vi "Q14070-Z060A - 副本.vi"() -> ()   [LabVIEW 2013]
uses:
  <vilib>/Utility/error.llb/whitespace.ctl
  <vilib>/Utility/file.llb/Read From Spreadsheet File (string).vi
  <vilib>/express/express arith-compare/Formula/XNode/ExpressFormulaBlockNode.xnode
  PCI8622_32.dll
  <vilib>/printing/EasyPrintingControls.llb/contents.ctl
  <vilib>/Utility/NIReport.llb/NI_ReportGenerationCore.lvlib
  <vilib>/printing/EasyPrintingControls.llb/report_type.ctl
  <vilib>/printing/EasyPrinting.llb/Easy Print VI Panel or Documentation (path).vi
  <vilib>/Utility/NIReport.llb/NI_report.lvclass
panel:
  out "最大轴向力标准(N)":dbl=200.0 caption="L+Lmax(mm)" format="%#.3f"
  out "右平均轴向力(N)":dbl caption="L+Lmax(mm)" format="%#.3f"
  out "左平均轴向力(N)":dbl caption="最大位移偏离Lmax(mm)" format="%#.3f"
  out "员工ID":string
  in  "机械间隙值":dbl=2.0
  out "急停":bool
  out "报警":dbl
  out "报警提示":string
  out "DeviceHandle":u32
  in  "设定轴向力调整次数":dbl=6.0
  out "出支线工步号":u32
  in  "最小间隙(mm)":dbl=0.001 format="%#.3f"
  in  "测头气缸右移":bool
  in  "测头气缸左移":bool
  in  "轴向力已做次数":dbl
  out "全行程间隙及轴向力合格":bool
  out "轴向力启动":bool
  out "间隙启动":bool
  in  "夹头松开":bool
  in  "夹头夹紧":bool
  out "找帽扭矩":dbl=8.0 caption="压力传感器" format="%#.2f"
  out "error out":errorcluster
  out "型号数量":i32
  out "error out 4":errorcluster
  in  "设定间隙调整次数":dbl=6.0
  out "读取产品ID":string
  out "下工位备料":bool
  out "下工位测试":bool
  out "下工位自动":bool
  out "下工位备料H":bool
  out "下工位测试H":bool
  out "下工位自动H":bool
  out "FGCS":string
  out "KSJJ":string
  out "Z060ARFID":string
  out "轴向力Y":dbl[](array[numeric])
  out "轴向力X":dbl[](array[numeric])
  out "间隙X数组":dbl[](array[numeric])
  out "间隙Y数组":dbl[](array[numeric])
  out "error out 3":errorcluster caption="错误输出"
  out "rfid工步号":u32
  out "芯片ID":string="201209190001"
  out "rfid完成":bool
  out "rfid触发":bool
  out "本序已做":bool
  in  "回零完成":bool
  in  "电动缸回零":bool
  in  "已调试次数":dbl
  in  "需调整角度(度)":dbl
  in  "转向器中心":dbl
  out "扭矩到达":bool
  out "黄灯":bool
  out "红灯":bool
  in  "基准位移":dbl caption="压力传感器" format="%#.3f"
  out "上序不合格":bool
  out "单点间隙合格":bool
  out "上序合格":bool
  out "测头机构电机":u32
  out "复位":bool
  in  "型号选择":u16(ring)=1 items=["J709", "J728", "J706"]
  in  "联线按钮":bool
  in  "工步号":u32
  in  "产品ID":string="201209190001"
  out "间隙位移(mm)":dbl caption="压力传感器" format="%#.3f"
  out "齿条推拉力(N)":dbl format="%#.2f"
  out "齿条扭矩(Nm)":dbl format="%#.2f"
  out "通讯状态":bool
  in  "员工ID":string
  out "员工姓名":string
  out "工步提示":string
  out "ADODB._Connection Out 2":refnum<k7>
  out "旋转齿条电机":u32
  out "电动缸电机":u32
  in  "停止":bool
  in  "参数加载":bool
  in  "选项卡控件":T1(tab)
  out "扭动曲线":cluster{"Y":dbl[], "Y":dbl[]}[](graph) caption="压球涨堵头1"
  out "中间位置间隙":dbl caption="间隙值L(mm)" format="%#.3f"
  in  "中间间隙标准(mm)":dbl=0.07 format="%#.3f"
  in  "找帽OK":bool
  in  "全行程180°外间隙标准(mm)":dbl=0.1 format="%#.3f"
  out "右180°外全行程间隙":dbl caption="正向最大间隙L1(mm)" format="%#.4f"
  out "左180°外全行程间隙":dbl caption="正向最大间隙L1(mm)" format="%#.4f"
  out "右180°内全行程间隙":dbl caption="正向最大间隙L1(mm)" format="%#.4f"
  out "左180°内全行程间隙":dbl caption="正向最大间隙L1(mm)" format="%#.4f"
  in  "全行程180°内间隙标准(mm)":dbl=0.07 format="%#.3f"
  out "左全行程间隙":dbl caption="正向最大间隙L1(mm)" format="%#.3f"
  out "右全行程间隙":dbl caption="正向最大间隙L1(mm)" format="%#.3f"
  out "总圈数最大值":dbl
  out "总圈数标准":dbl
  out "总行程最大值":dbl
  out "总行程标准(mm)":dbl
  out "平均轴向力MAX(N)":dbl=200.0 caption="L+Lmax(mm)" format="%#.3f"
  out "力波动标准(N)":dbl=60.0 caption="L+Lmax(mm)" format="%#.3f"
  out "轴向力标准(N)":dbl=100.0 caption="L+Lmax(mm)" format="%#.3f"
  out "右最大轴向力(N)":dbl caption="L+Lmax(mm)" format="%#.3f"
  out "左轴向力波动(N)":dbl caption="最大位移偏离Lmax(mm)" format="%#.3f"
  out "左最大轴向力(N)":dbl caption="最大位移偏离Lmax(mm)" format="%#.3f"
  out "行程跳动曲线":cluster{"Y":dbl[], "Y":dbl[]}[](graph) caption="压球涨堵头1"
  out "右轴向力波动(N)":dbl format="%#.3f"
  out "总行程(mm)":dbl format="%#.2f"
  out "总圈数":dbl format="%#.2f"
  in  "不合格品":bool
  in  "扭矩停止值":dbl=16.0
  in  "齿条右极限":dbl=-70.0 caption="压力传感器" format="%#.2f"
  in  "齿条左极限":dbl=-262.0 caption="压力传感器" format="%#.2f"
  in  "齿条移动速度":dbl=5.0 caption="压力传感器" format="%#.2f"
  in  "旋转伺服找帽转速":dbl=5.0 caption="压力传感器" format="%#.2f"
  in  "测量点扭矩":dbl=4.0 caption="压力传感器" format="%#.2f"
  in  "旋转伺服测量转速":dbl caption="压力传感器" format="%#.2f"
  in  "测头机构轴后退位":dbl=30.0 caption="压力传感器" format="%#.2f"
  in  "测头机构轴待检位":dbl caption="压力传感器" format="%#.2f"
  in  "测头机构轴检测位":dbl caption="压力传感器" format="%#.2f"
  in  "测头机构轴移动速度":dbl caption="压力传感器" format="%#.2f"
  in  "全行程修正":dbl=5.5
  out "点胶":bool
  in  "夹头松开":bool
  in  "夹头夹紧":bool
  in  "测头气缸右移":bool
  in  "测头气缸左移":bool
  in  "支线下降":bool
  in  "支线顶升":bool
  in  "出支线":bool
  in  "进支线":bool
  in  "主线下降":bool
  in  "主线顶升":bool
  in  "下阻挡器放行":bool
  in  "上阻挡器放行":bool
  out "夹头夹紧位":bool
  out "测头左位":bool
  out "测头右位":bool
  out "夹头松开":bool
  out "记号笔":bool
  in  "测头机构轴使能":bool
  in  "测头机构轴后退":bool
  in  "测头机构轴前进":bool
  in  "电动缸速度(mm/s)":dbl=10.0 format="%#.3f"
  out "电动缸位置(mm)":dbl=10000.0 format="%#.3f"
  in  "旋转伺服速度(°/s)":dbl=10.0 format="%#.3f"
  out "旋转伺服位置(°)":dbl=10000.0 format="%#.3f"
  in  "测头机构轴速度(mm/s)":dbl=10.0 format="%#.3f"
  out "测头机构轴位置(mm)":dbl=10000.0 format="%#.3f"
  in  "旋转齿条轴右转":bool
  in  "旋转齿条轴左转":bool
  in  "旋转齿条轴使能":bool
  in  "电动缸后退":bool
  in  "电动缸使能":bool
  in  "电动缸前进":bool
  in  "齿条扭矩比例偏移":dbl=1.0 format="%#.2f"
  in  "齿条扭矩零点偏移":dbl format="%#.2f"
  in  "齿条推拉力比例偏移":dbl=1.0 format="%#.2f"
  in  "齿条推拉力零点偏移":dbl format="%#.2f"
  in  "间隙位移比例偏移":dbl=1.0 format="%#.2f"
  in  "间隙位移零点偏移":dbl format="%#.2f"
  in  "传感器参数保存":bool
  in  "参数修改":bool
  in  "参数查询":bool
  in  "参数浏览表":string[][](table)
  # "芜湖机械转向器装配线"
  # "间隙及轴向力检测"
  # "Q14070机械转向器装配线"
  # "湖北唯思凌科装备制造有限公司 设计开发 (C)2015"
  # "≤"
  # "间隙测量判定值"
  # "间隙测量结果"
  # "≤"
  # "≤"
  # "≤"
  # "轴向力测量结果"
  # "轴向力测量标准"
  # "≤"
  # "≥"
  # "≤"
  # "≥"
  # "≤"
  # "≥"
  # "≤"
  # "不得大于20NM"
  # "传感器校验区"
  # "关于传感器校验：\n1、传感器校验需要由具备资质的单位或部门进行校验。\n2、具备权限的用户才能够修改传感器校验参数和试验参数。\n3、修改校验参数方法：先将比例偏移置为1，修改零点偏移，使零点值与校验的传感器一致；然后根据增幅调整比例偏移。"
  # "注意：\n具备权限的用户才能够修改传感器校验参数和试验参数！"
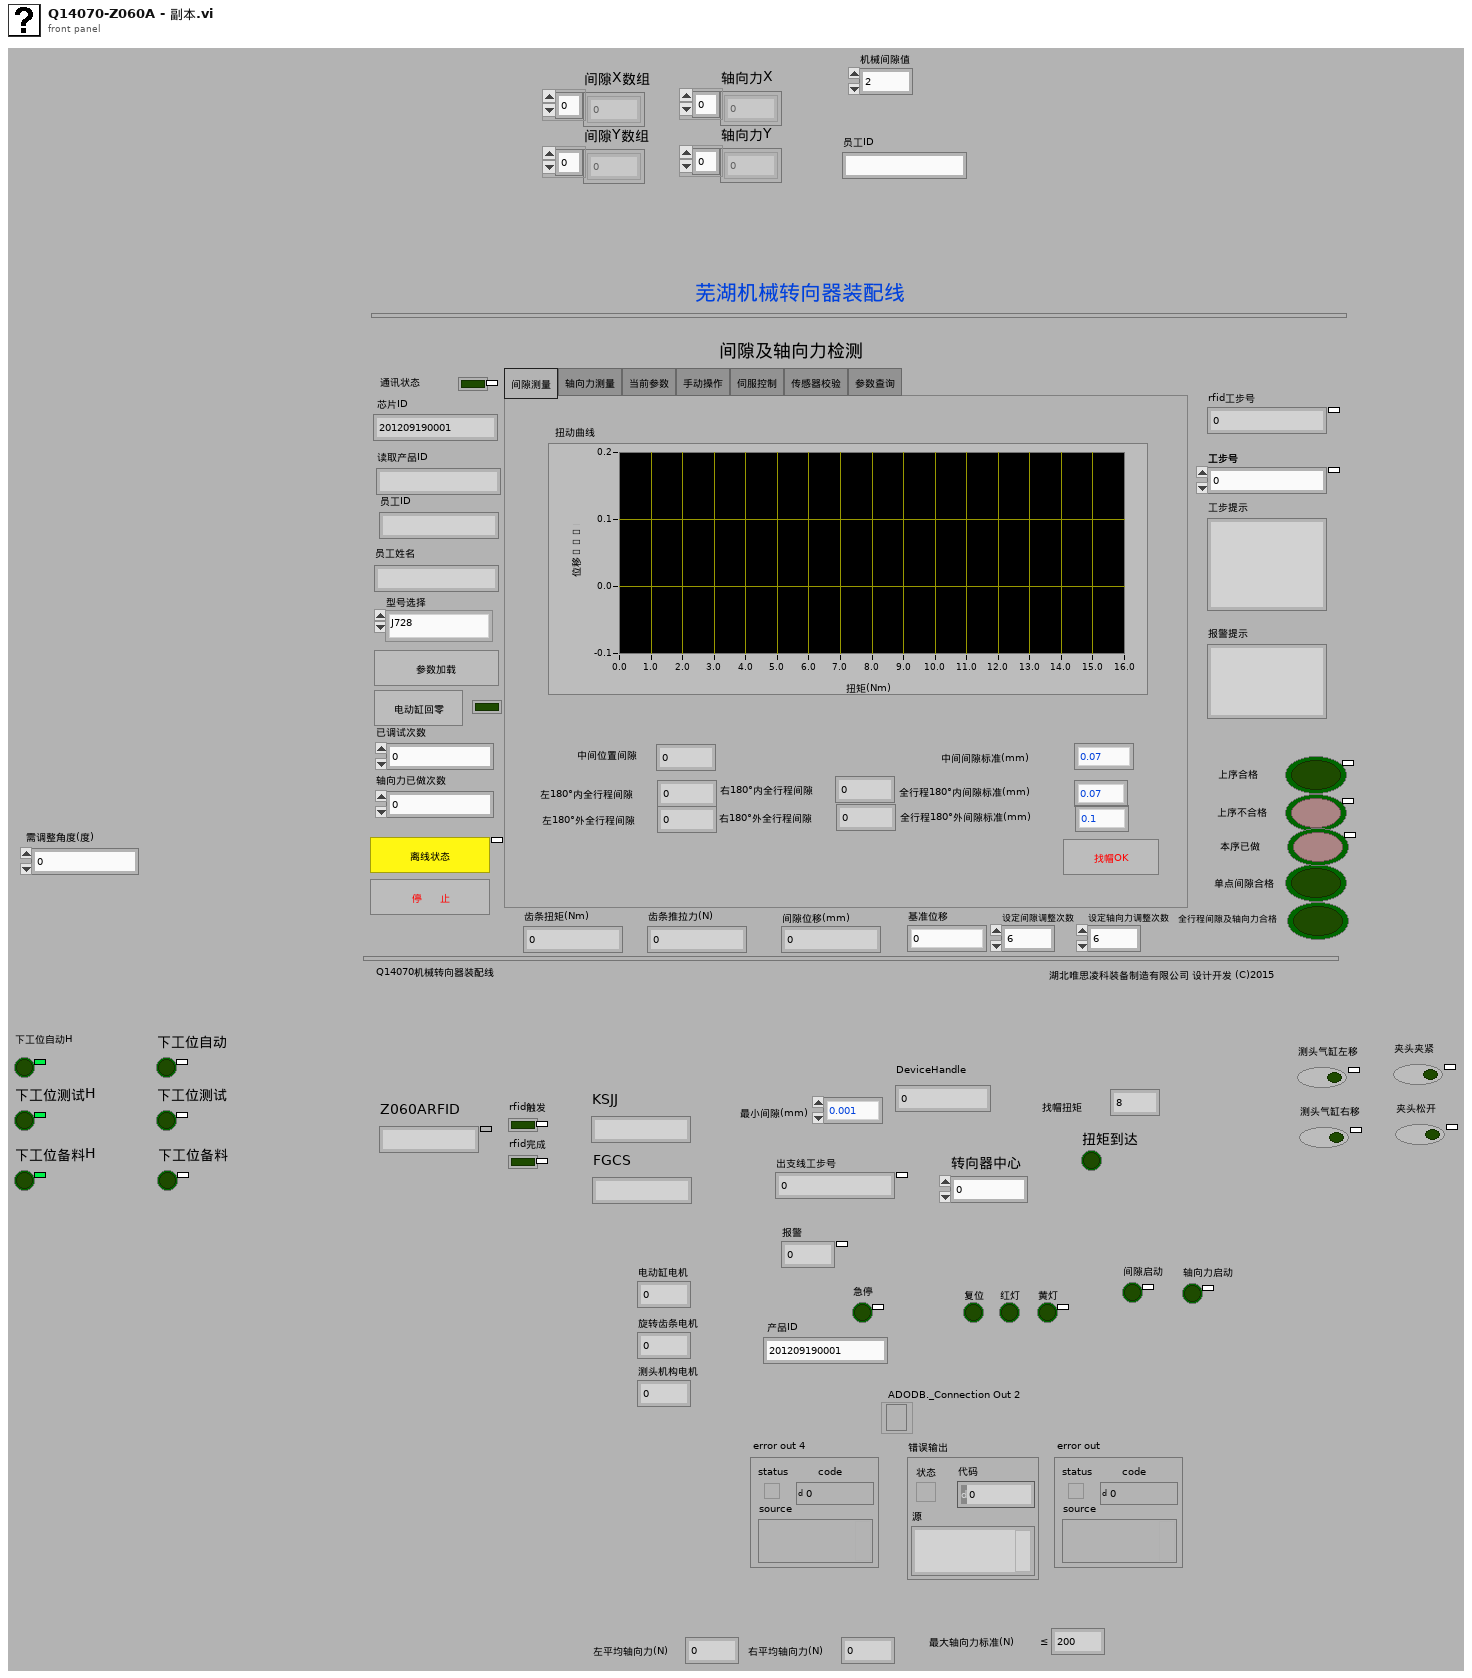
[diagram p1: front panel]
types:
  T1 = enum32{"间隙测量", "轴向力测量", "当前参数", "手动操作", "伺服控制", "传感器校验", "参数查询"}
  T2 = typedef "NI_ReportGenerationCore.lvlib/report_type.ctl" = u16
  T3 = typedef "NI_ReportGenerationCore.lvlib/contents.ctl" = u16
  T4 = typedef "imagedata.ctl" = cluster{"image type":i32, "image depth":i32, "image":u8[], "mask":u8[], "colors":u32[], "Rectangle":cluster{"left":i16, "top":i16, "right":i16, "bottom":i16}}
  T5 = enum8{"Enabled", "Disabled", "Disabled and Grayed Out"}
  T6 = typedef "whitespace.ctl" = u16
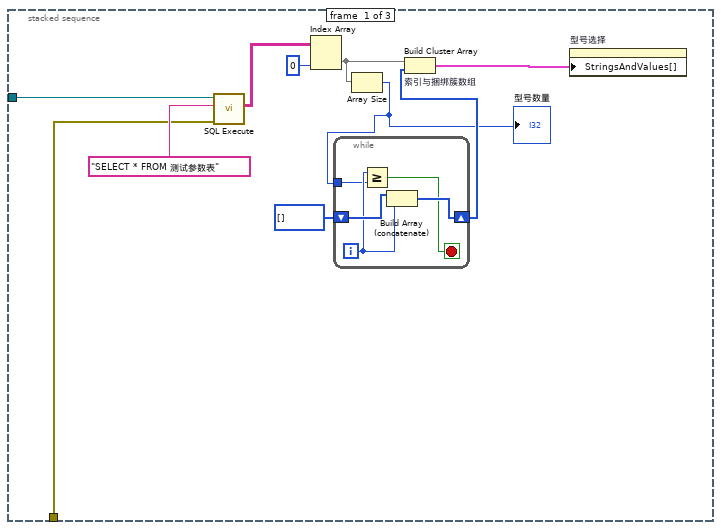
[diagram p4: hidden frame]
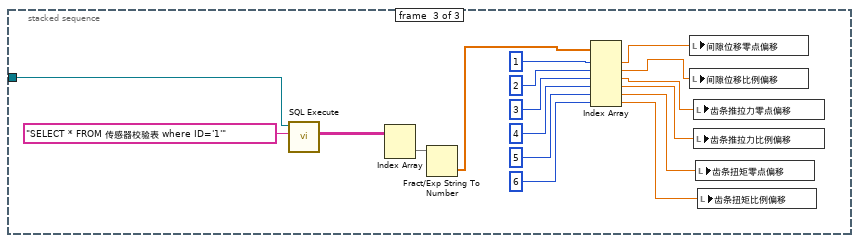
[diagram p5: hidden frame]
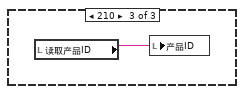
[diagram p7: hidden frame]
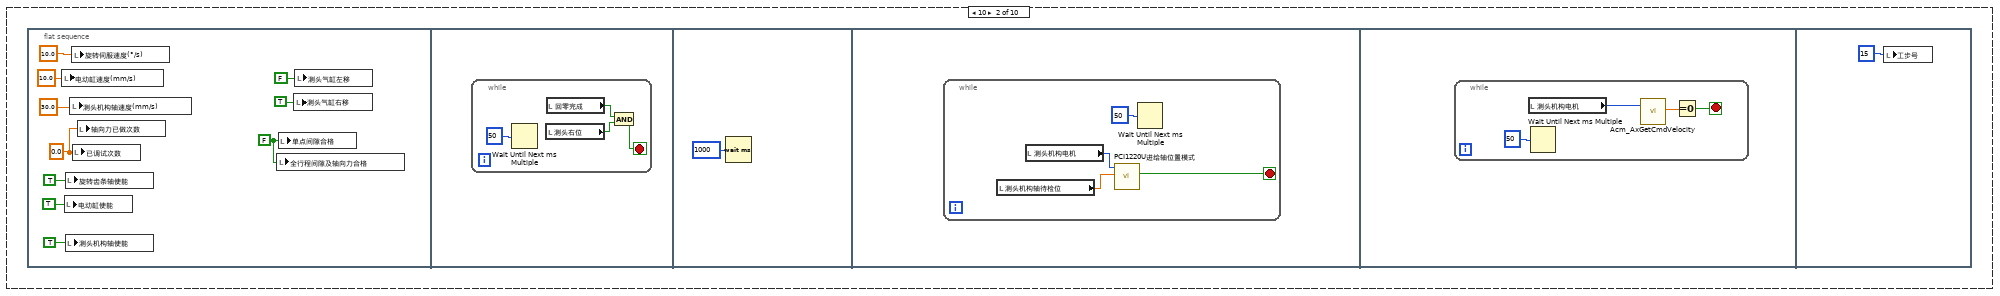
[diagram p9: hidden frame]
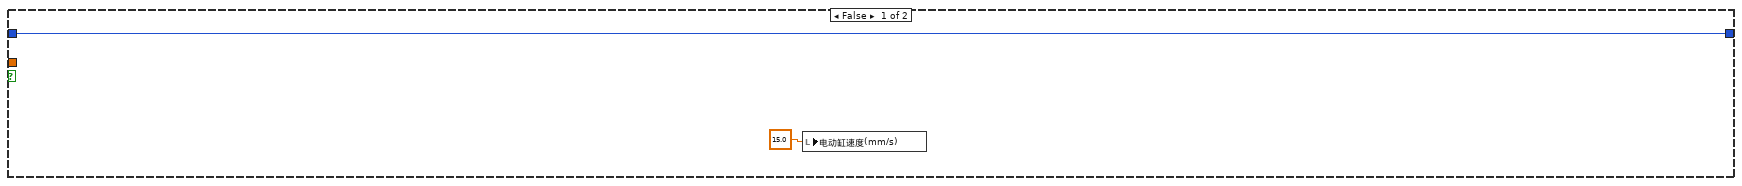
[diagram p10: hidden frame]
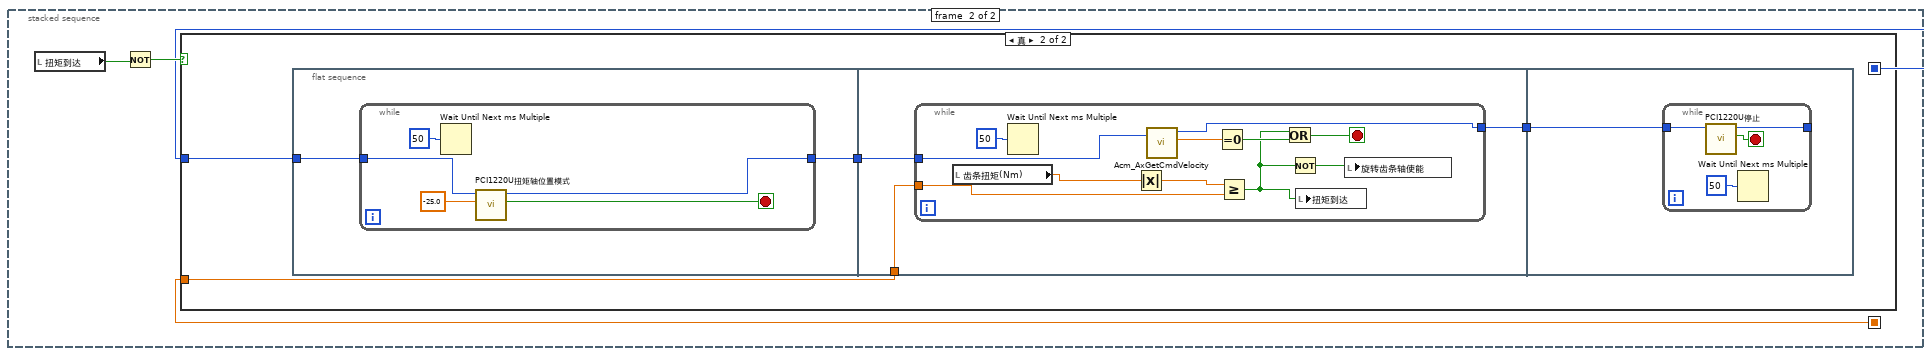
[diagram p11: hidden frame]
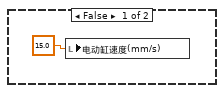
[diagram p12: hidden frame]
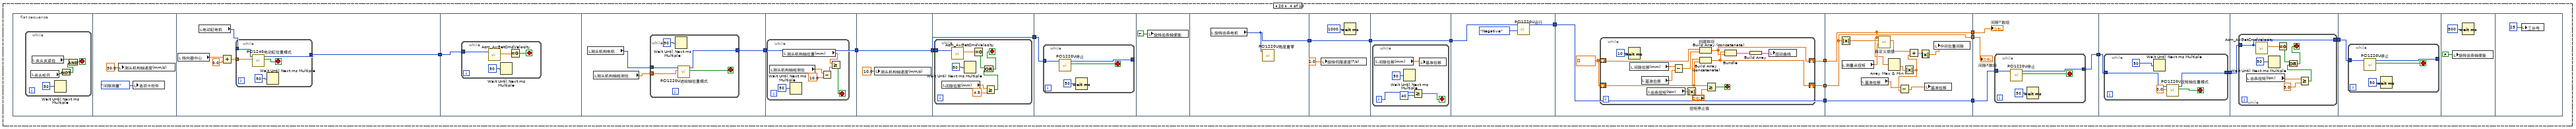
[diagram p14: hidden frame]
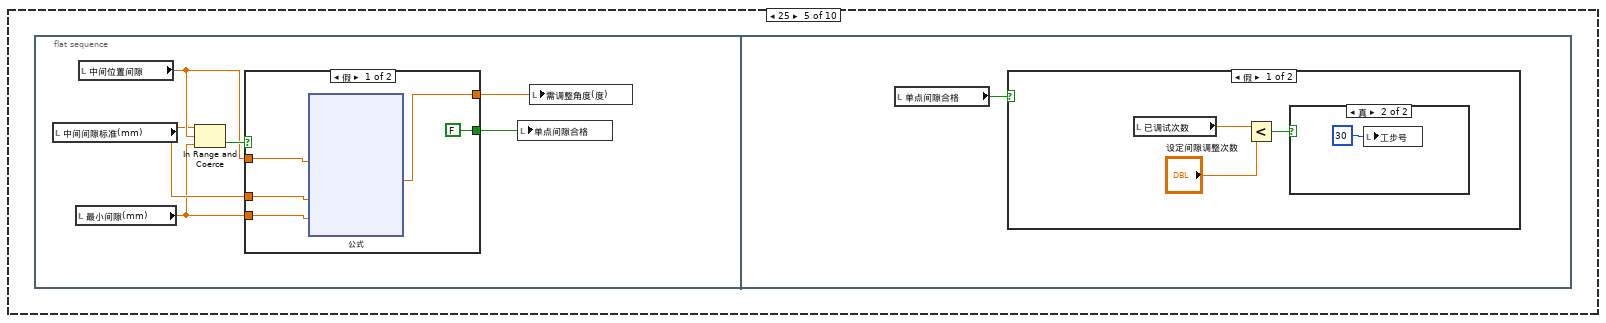
[diagram p15: hidden frame]
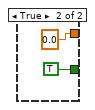
[diagram p16: hidden frame]
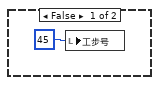
[diagram p17: hidden frame]
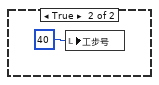
[diagram p18: hidden frame]
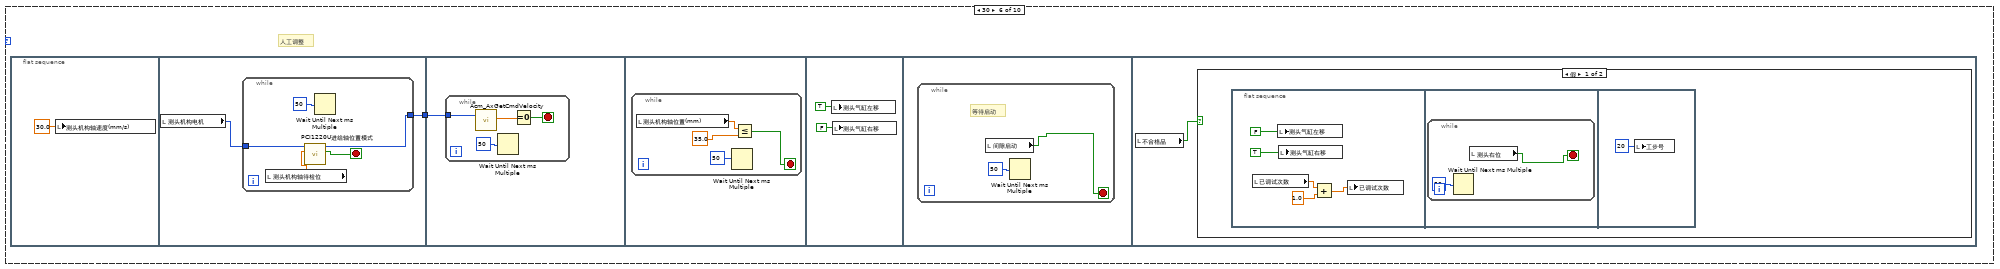
[diagram p19: hidden frame]
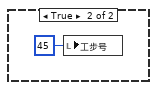
[diagram p20: hidden frame]
diagram:
  n1 = while {
    stop <- w7 stop-if-true
    n2 = local read "工步号"() -> (w5:u32)
    n3 = case shown="15" w5 {
      frame 0, Default {
      }
      frame 10 {
        n4 = flat-sequence {
          frame #0 {
            w8 = FALSE ("单点间隙合格")
            w9 = 0.0 ("已调试次数")
            n5 = local write "电动缸速度(mm/s)"(10.0 ("电动缸速度(mm/s)")) -> ()
            n6 = local write "电动缸使能"(TRUE ("电动缸使能")) -> ()
            n7 = local write "旋转齿条轴使能"(TRUE ("旋转齿条轴使能")) -> ()
            n8 = local write "测头机构轴使能"(TRUE ("调整机构轴使能")) -> ()
            n9 = local write "测头机构轴速度(mm/s)"(30.0 ("调整机构轴速度(mm/s)")) -> ()
            n10 = local write "旋转伺服速度(°/s)"(10.0 ("旋转齿条轴速度(°/s)")) -> ()
            n11 = local write "已调试次数"(w9) -> ()
            n12 = local write "轴向力已做次数"(w9) -> ()
            n13 = local write "全行程间隙及轴向力合格"(w8) -> ()
            n14 = local write "单点间隙合格"(w8) -> ()
            n15 = local write "测头气缸右移"(TRUE ("测头气缸右移")) -> ()
            n16 = local write "测头气缸左移"(FALSE ("测头气缸左移")) -> ()
          }
          frame #1 {
            n17 = while {
              stop <- w18 stop-if-true
              n18 = Wait Until Next ms Multiple(millisecond multiple=u32 50 ("毫秒倍数")) -> ()  [unwired: 1 out]
              n19 = local read "测头右位"() -> (w19:bool)
              n20 = local read "回零完成"() -> (w20:bool)
              n21 = And(x=w20, y=w19) -> (x .and. y?=w18:bool)
            }
          }
          frame #2 {
            n22 = Wait (ms)(milliseconds to wait=u32 1000 ("等待时间（毫秒）")) -> ()  [unwired: 1 out]
          }
          frame #3 {
            n23 = while {
              stop <- w26 stop-if-true
              n24 = local read "测头机构轴待检位"() -> (w23:dbl)
              n25 = local read "测头机构电机"() -> (w24:u32)
              n26 = call "PCI1220U进给轴位置模式.vi"("Distance"=w23, "AxisHandle IN"=w24) -> ("AbsSuccess"=w26:bool)  [unwired: 8 in, 1 out]
              n27 = Wait Until Next ms Multiple(millisecond multiple=u32 50 ("毫秒倍数")) -> ()  [unwired: 1 out]
            }
          }
          frame #4 {
            n28 = while {
              stop <- w29 stop-if-true
              n29 = local read "测头机构电机"() -> (w27:u32)
              n30 = Wait Until Next ms Multiple(millisecond multiple=u32 50 ("毫秒倍数")) -> ()  [unwired: 1 out]
              n31 = call <userlib>:"Acm_AxGetCmdVelocity.vi"("AxisHandle"=w27) -> ("Velocity"=w30:dbl)  [unwired: 1 in, 3 out]
              n32 = Equal To 0?(x=w30) -> (x = 0?=w29:bool)
            }
          }
          frame #5 {
            n33 = local write "工步号"(u32 15 ("工步号")) -> ()
          }
        }
      }
      frame 15 {
        n34 = flat-sequence {
          tunnel: [w42] -> w33
          tunnel: w33 -> [w144]
          tunnel: [w144] -> w34
          tunnel: [w149] -> w37
          tunnel: ["转向器中心"] -> w36
          tunnel: w34 -> [w149]
          tunnel: w37 -> [w158]
          tunnel: w36 -> [w157]
          tunnel: [w156] -> w35
          tunnel: w35 -> [w165]
          tunnel: [w164] -> w32
          tunnel: w32 -> [w176]
          frame #0 {
            n35 = local write "扭矩到达"(FALSE ("扭矩到达")) -> ()
            n36 = local write "旋转伺服速度(°/s)"(10.0 ("旋转齿条轴速度(°/s)")) -> ()
            "找帽扭矩" <- 8.0 ("找帽扭矩")
          }
          frame #1 {
            n37 = Wait Until Next ms Multiple(millisecond multiple=u32 50 ("毫秒倍数")) -> ()  [unwired: 1 out]
            n38 = while {
              stop <- w45 stop-if-true
              n39 = stacked-sequence {
                seq-local: [w47 _] -> [_ w88]
                seq-local: [w51 _] -> [_ w87]
                frame #0 {
                  n40 = local read "扭矩到达"() -> (w49:bool)
                  n41 = local read "找帽扭矩"() -> (w47:dbl)
                  n42 = local read "旋转齿条电机"() -> (w48:u32)
                  n43 = Not(x=w49) -> (.not. x?=w50:bool)
                  n44 = case shown="真" w50 {
                    tunnel: [w53 w54] -> w51
                    tunnel: w48 -> [w53 w58]
                    tunnel: w47 -> [_ w56]
                    frame False {
                      n45 = local write "电动缸速度(mm/s)"(15.0 ("电动缸速度(mm/s)")) -> ()
                    }
                    frame True {
                      n46 = flat-sequence {
                        tunnel: w58 -> [w60]
                        tunnel: [w59] -> w57
                        tunnel: w57 -> [w68]
                        tunnel: w56 -> [w67]
                        tunnel: [w66] -> w55
                        tunnel: w55 -> [w81]
                        tunnel: [w80] -> w54
                        frame #0 {
                          n47 = while {
                            tunnel: [w64] -> w59
                            tunnel: w60 -> [w61]
                            stop <- w63 stop-if-true
                            n48 = Wait Until Next ms Multiple(millisecond multiple=u32 50 ("毫秒倍数")) -> ()  [unwired: 1 out]
                            n49 = call "PCI1220U扭矩轴位置模式.vi"("Distance"=13.0, "AxisHandle IN"=w61) -> ("AbsSuccess"=w63:bool, "AxisHandle OUT"=w64:u32)  [unwired: 8 in]
                          }
                        }
                        frame #1 {
                          n50 = while {
                            tunnel: w68 -> [w78]
                            tunnel: w67 -> [w73]
                            tunnel: [w72] -> w66
                            stop <- w74 stop-if-true
                            n51 = local read "齿条扭矩(Nm)"() -> (w71:dbl)
                            n52 = Wait Until Next ms Multiple(millisecond multiple=u32 10 ("毫秒倍数")) -> ()  [unwired: 1 out]
                            n53 = Absolute Value(x=w71) -> (abs(x)=w76:dbl)
                            n54 = call <userlib>:"Acm_AxGetCmdVelocity.vi"("AxisHandle"=w78) -> ("Velocity"=w77:dbl, "AxisHandle"=w72:u32)  [unwired: 1 in, 2 out]
                            n55 = Equal To 0?(x=w77) -> (x = 0?=w75:bool)
                            n56 = Greater Or Equal?(x=w76, y=w73) -> (x >= y?=w70:bool)
                            n57 = Or "或"(x=w70, y=w75) -> (x .or. y?=w74:bool)
                            n58 = local write "扭矩到达"(w70) -> ()
                            n59 = Not(x=w70) -> (.not. x?=w69:bool)
                            n60 = local write "旋转齿条轴使能"(w69) -> ()
                          }
                        }
                        frame #2 {
                          n61 = while {
                            tunnel: w81 -> [w85]
                            tunnel: [w82] -> w80
                            stop <- w84 stop-if-true
                            n62 = call "PCI1220U停止.vi"("AxisHandle IN"=w85) -> ("完成"=w84:bool, "AxisHandle OUT"=w82:u32)  [unwired: 9 in]
                            n63 = Wait Until Next ms Multiple(millisecond multiple=u32 50 ("毫秒倍数")) -> ()  [unwired: 1 out]
                          }
                        }
                      }
                    }
                  }
                }
                frame #1 {
                  n64 = local read "扭矩到达"() -> (w86:bool)
                  n65 = Not(x=w86) -> (.not. x?=w89:bool)
                  n66 = case shown="真" w89 {
                    tunnel: w87 -> [_ w94]
                    tunnel: w88 -> [_ w92]
                    frame False {
                      n67 = local write "电动缸速度(mm/s)"(15.0 ("电动缸速度(mm/s)")) -> ()
                    }
                    frame True {
                      n68 = flat-sequence {
                        tunnel: w94 -> [w95]
                        tunnel: [w96] -> w93
                        tunnel: w93 -> [w104]
                        tunnel: w92 -> [w103]
                        tunnel: [w102] -> w91
                        tunnel: w91 -> [w116]
                        frame #0 {
                          n69 = while {
                            tunnel: [w100] -> w96
                            tunnel: w95 -> [w97]
                            stop <- w99 stop-if-true
                            n70 = Wait Until Next ms Multiple(millisecond multiple=u32 50 ("毫秒倍数")) -> ()  [unwired: 1 out]
                            n71 = call "PCI1220U扭矩轴位置模式.vi"("Distance"=-25.0, "AxisHandle IN"=w97) -> ("AbsSuccess"=w99:bool, "AxisHandle OUT"=w100:u32)  [unwired: 8 in]
                          }
                        }
                        frame #1 {
                          n72 = while {
                            tunnel: w104 -> [w114]
                            tunnel: [w109] -> w102
                            tunnel: w103 -> [w108]
                            stop <- w110 stop-if-true
                            n73 = local read "齿条扭矩(Nm)"() -> (w107:dbl)
                            n74 = Wait Until Next ms Multiple(millisecond multiple=u32 50 ("毫秒倍数")) -> ()  [unwired: 1 out]
                            n75 = Absolute Value(x=w107) -> (abs(x)=w112:dbl)
                            n76 = call <userlib>:"Acm_AxGetCmdVelocity.vi"("AxisHandle"=w114) -> ("Velocity"=w113:dbl, "AxisHandle"=w109:u32)  [unwired: 1 in, 2 out]
                            n77 = Equal To 0?(x=w113) -> (x = 0?=w111:bool)
                            n78 = Greater Or Equal?(x=w112, y=w108) -> (x >= y?=w105:bool)
                            n79 = Or(x=w105, y=w111) -> (x .or. y?=w110:bool)
                            n80 = Not(x=w105) -> (.not. x?=w106:bool)
                            n81 = local write "扭矩到达"(w105) -> ()
                            n82 = local write "旋转齿条轴使能"(w106) -> ()
                          }
                        }
                        frame #2 {
                          n83 = while {
                            tunnel: w116 -> [w120]
                            tunnel: [w117] -> _
                            stop <- w119 stop-if-true
                            n84 = call "PCI1220U停止.vi"("AxisHandle IN"=w120) -> ("完成"=w119:bool, "AxisHandle OUT"=w117:u32)  [unwired: 9 in]
                            n85 = Wait Until Next ms Multiple(millisecond multiple=u32 50 ("毫秒倍数")) -> ()  [unwired: 1 out]
                          }
                        }
                      }
                    }
                  }
                }
              }
              n86 = Wait Until Next ms Multiple(millisecond multiple=u32 50 ("毫秒倍数")) -> ()  [unwired: 1 out]
              n87 = local read "扭矩到达"() -> (w45:bool)
            }
            n88 = flat-sequence {
              tunnel: [w122] -> w44
              tunnel: w44 -> [w128]
              tunnel: [w128] -> w41
              tunnel: [w137] -> w42
              tunnel: w41 -> [w137]
              frame #0 {
                n89 = local write "电动缸速度(mm/s)"(5.0 ("电动缸速度(mm/s)")) -> ()
              }
              frame #1 {
                n90 = while {
                  tunnel: [w126] -> w122
                  stop <- w125 stop-if-true
                  n91 = local read "齿条左极限"() -> (w123:dbl)
                  n92 = local read "电动缸电机"() -> (w127:u32)
                  n93 = Wait Until Next ms Multiple(millisecond multiple=u32 50 ("毫秒倍数")) -> ()  [unwired: 1 out]
                  n94 = call "PCI1240电动缸位置模式 .vi"("Distance"=w123, "AxisHandle IN"=w127) -> ("AbsSuccess"=w125:bool, "AxisHandle OUT"=w126:u32)  [unwired: 8 in]
                }
              }
              frame #2 {
                n95 = while {
                  tunnel: w128 -> [w135]
                  stop <- w132 stop-if-true
                  n96 = local read "齿条推拉力(N)"() -> (w131:dbl)
                  n97 = call <userlib>:"Acm_AxGetCmdVelocity.vi"("AxisHandle"=w135) -> ("Velocity"=w136:dbl)  [unwired: 1 in, 3 out]
                  n98 = Wait Until Next ms Multiple(millisecond multiple=u32 50 ("毫秒倍数")) -> ()  [unwired: 1 out]
                  n99 = Less Or Equal?(x=w131, y=-1000.0) -> (x <= y?=w129:bool)
                  n100 = Equal To 0?(x=w136) -> (x = 0?=w133:bool)
                  n101 = Or(x=w133, y=w129) -> (x .or. y?=w132:bool)
                }
              }
              frame #3 {
                n102 = while {
                  tunnel: w137 -> [w141]
                  tunnel: [w138] -> _
                  stop <- w140 stop-if-true
                  n103 = call "PCI1220U停止.vi"("AxisHandle IN"=w141) -> ("完成"=w140:bool, "AxisHandle OUT"=w138:u32)  [unwired: 9 in]
                  n104 = Wait Until Next ms Multiple(millisecond multiple=u32 50 ("毫秒倍数")) -> ()  [unwired: 1 out]
                }
              }
            }
          }
          frame #2 {
            n105 = while {
              stop <- "找帽OK" stop-if-true
              n106 = Wait Until Next ms Multiple(millisecond multiple=u32 50 ("毫秒倍数")) -> ()  [unwired: 1 out]
            }
            n107 = Wait Until Next ms Multiple(millisecond multiple=u32 500 ("毫秒倍数")) -> ()  [unwired: 1 out]
            n108 = local write "夹头夹紧"(TRUE ("夹头夹紧")) -> ()
            n109 = local write "夹头松开"(FALSE ("夹头松开")) -> ()
          }
          frame #3 {
            n110 = disable-structure shown="禁用" {
              disable-tunnel: [w153 _] -> _
              frame Disabled {
                n111 = local read "齿条右极限"() -> (w151:dbl)
                n112 = local read "齿条左极限"() -> (w152:dbl)
                n113 = Add(x=w152, y=w151) -> (x+y=w155:dbl)
                n114 = Divide(x=w155, y=2.0) -> (x/y=w153:dbl)
              }
              frame Enabled {
              }
            }
            n115 = local write "电动缸速度(mm/s)"(15.0 ("电动缸轴移动速度")) -> ()
          }
          frame #4 {
            n116 = while {
              tunnel: w158 -> [w163]
              tunnel: w157 -> [w162]
              tunnel: [w159] -> w156
              stop <- w161 stop-if-true
              n117 = call "PCI1240电动缸位置模式 .vi"("Distance"=w162, "AxisHandle IN"=w163) -> ("AbsSuccess"=w161:bool, "AxisHandle OUT"=w159:u32)  [unwired: 8 in]
              n118 = Wait Until Next ms Multiple(millisecond multiple=u32 50 ("毫秒倍数")) -> ()  [unwired: 1 out]
            }
          }
          frame #5 {
            n119 = while {
              tunnel: w165 -> [w175]
              tunnel: [w166] -> w164
              stop <- w167 stop-if-true
              n120 = local read "齿条推拉力(N)"() -> (w172:dbl)
              n121 = call <userlib>:"Acm_AxGetCmdVelocity.vi"("AxisHandle"=w175) -> ("Velocity"=w174:dbl, "AxisHandle"=w166:u32)  [unwired: 1 in, 2 out]
              n122 = Wait Until Next ms Multiple(millisecond multiple=u32 50 ("毫秒倍数")) -> ()  [unwired: 1 out]
              n123 = Equal To 0?(x=w174) -> (x = 0?=w169:bool)
              n124 = Absolute Value(x=w172) -> (abs(x)=w171:dbl)
              n125 = Greater Or Equal?(x=w171, y=1000.0) -> (x >= y?=w168:bool)
              n126 = Or(x=w169, y=w168) -> (x .or. y?=w167:bool)
            }
          }
          frame #6 {
            n127 = while {
              tunnel: w176 -> [w180]
              tunnel: [w179] -> _
              stop <- w178 stop-if-true
              n128 = call "PCI1220U停止.vi"("AxisHandle IN"=w180) -> ("完成"=w178:bool, "AxisHandle OUT"=w179:u32)  [unwired: 9 in]
              n129 = Wait (ms)(milliseconds to wait=u32 50 ("毫秒倍数")) -> ()  [unwired: 1 out]
            }
          }
          frame #7 {
            n130 = local write "工步号"(u32 20 ("工步号")) -> ()
          }
        }
      }
      frame 20 {
        n131 = flat-sequence {
          tunnel: [w211] -> w192
          tunnel: w192 -> [w217]
          tunnel: [w223] -> w184
          tunnel: w184 -> [w230]
          tunnel: [w230] -> w183
          tunnel: w183 -> [w238]
          tunnel: [w238] -> w182
          tunnel: w182 -> [w239]
          tunnel: [w239] -> w191
          tunnel: w191 -> [w248]
          tunnel: [w254] -> w189
          tunnel: [w256] -> w190
          tunnel: w189 -> [w256]
          tunnel: [w258] -> w185
          tunnel: w190 -> [w258]
          tunnel: w185 -> [w265]
          tunnel: [w264] -> w196
          tunnel: [w269] -> w195
          tunnel: [w268] -> w194
          tunnel: w196 -> [w267]
          tunnel: [w267] -> w193
          tunnel: [w296] -> w199
          tunnel: [w293] -> w198
          tunnel: w195 -> [w293]
          tunnel: [w292] -> w197
          tunnel: w194 -> [w292]
          tunnel: w193 -> [w296]
          tunnel: w199 -> [w300]
          tunnel: [w299] -> w188
          tunnel: w198 -> [w297]
          tunnel: w197 -> [w298]
          tunnel: w188 -> [w306]
          tunnel: [w305] -> w187
          tunnel: w187 -> [w313]
          tunnel: [w312] -> w186
          tunnel: w186 -> [w322]
          frame #0 {
            n132 = while {
              stop <- w202 stop-if-true
              n133 = local read "夹头松开"() -> (w203:bool)
              n134 = local read "夹头夹紧位"() -> (w201:bool)
              n135 = Wait Until Next ms Multiple(millisecond multiple=u32 50 ("毫秒倍数")) -> ()  [unwired: 1 out]
              n136 = Not(x=w203) -> (.not. x?=w200:bool)
              n137 = And(x=w201, y=w200) -> (x .and. y?=w202:bool)
            }
          }
          frame #1 {
            n138 = local write "测头机构轴速度(mm/s)"(30.0 ("测头机构轴速度(mm/s)")) -> ()
            n139 = local write "选项卡控件"(T1."间隙测量" ("选项卡控件")) -> ()
          }
          frame #2 {
            n140 = local read "转向器中心"() -> (w209:dbl)
            n141 = local read "电动缸电机"() -> (w210:u32)
            n142 = Add(x=w209, y=0.0) -> (x+y=w208:dbl)
            n143 = while {
              tunnel: w210 -> [w216]
              tunnel: w208 -> [w215]
              tunnel: [w212] -> w211
              stop <- w214 stop-if-true
              n144 = call "PCI1240电动缸位置模式 .vi"("Distance"=w215, "AxisHandle IN"=w216) -> ("AbsSuccess"=w214:bool, "AxisHandle OUT"=w212:u32)  [unwired: 8 in]
              n145 = Wait Until Next ms Multiple(millisecond multiple=u32 50 ("毫秒倍数")) -> ()  [unwired: 1 out]
            }
          }
          frame #3 {
            n146 = while {
              tunnel: w217 -> [w221]
              stop <- w219 stop-if-true
              n147 = call <userlib>:"Acm_AxGetCmdVelocity.vi"("AxisHandle"=w221) -> ("Velocity"=w220:dbl)  [unwired: 1 in, 3 out]
              n148 = Wait Until Next ms Multiple(millisecond multiple=u32 50 ("毫秒倍数")) -> ()  [unwired: 1 out]
              n149 = Equal To 0?(x=w220) -> (x = 0?=w219:bool)
            }
          }
          frame #4 {
            n150 = local read "测头机构电机"() -> (w224:u32)
            n151 = local read "测头机构轴检测位"() -> (w222:dbl)
            n152 = while {
              tunnel: w224 -> [w227]
              tunnel: w222 -> [w226]
              tunnel: [w225] -> w223
              stop <- w229 stop-if-true
              n153 = Wait Until Next ms Multiple(millisecond multiple=u32 50 ("毫秒倍数")) -> ()  [unwired: 1 out]
              n154 = call "PCI1220U进给轴位置模式.vi"("Distance"=w226, "AxisHandle IN"=w227) -> ("AbsSuccess"=w229:bool, "AxisHandle OUT"=w225:u32)  [unwired: 8 in]
            }
          }
          frame #5 {
            n155 = while {
              stop <- w231 stop-if-true
              n156 = local read "测头机构轴检测位"() -> (w235:dbl)
              n157 = local read "测头机构轴位置(mm)"() -> (w234:dbl)
              n158 = Wait Until Next ms Multiple(millisecond multiple=u32 50 ("毫秒倍数")) -> ()  [unwired: 1 out]
              n159 = Subtract(x=w235, y=10.0) -> (x-y=w232:dbl)
              n160 = Greater Or Equal?(x=w234, y=w232) -> (x >= y?=w231:bool)
            }
          }
          frame #6 {
            n161 = local write "测头机构轴速度(mm/s)"(10.0 ("测头机构轴速度(mm/s)")) -> ()
          }
          frame #7 {
            n162 = while {
              tunnel: w239 -> [w247]
              stop <- w241 stop-if-true
              n163 = local read "间隙位移(mm)"() -> (w244:dbl)
              n164 = call <userlib>:"Acm_AxGetCmdVelocity.vi"("AxisHandle"=w247) -> ("Velocity"=w246:dbl)  [unwired: 1 in, 3 out]
              n165 = Wait Until Next ms Multiple(millisecond multiple=u32 50 ("毫秒倍数")) -> ()  [unwired: 1 out]
              n166 = Equal To 0?(x=w246) -> (x = 0?=w242:bool)
              n167 = Greater Or Equal?(x=w244, y=4.5) -> (x >= y?=w240:bool)
              n168 = Or(x=w242, y=w240) -> (x .or. y?=w241:bool)
            }
          }
          frame #8 {
            n169 = while {
              tunnel: w248 -> [w252]
              tunnel: [w251] -> _
              stop <- w250 stop-if-true
              n170 = call "PCI1220U停止.vi"("AxisHandle IN"=w252) -> ("完成"=w250:bool, "AxisHandle OUT"=w251:u32)  [unwired: 9 in]
              n171 = Wait (ms)(milliseconds to wait=u32 50 ("毫秒倍数")) -> ()  [unwired: 1 out]
            }
          }
          frame #9 {
            n172 = local write "旋转齿条轴使能"(TRUE ("旋转齿条轴使能")) -> ()
          }
          frame #10 {
            n173 = local read "旋转齿条电机"() -> (w254:u32)
            n174 = call "PCI1220U角度置零.vi"("AxisHandle IN"=w254) -> ()  [unwired: 10 in, 1 out]
          }
          frame #11 {
            n175 = local write "旋转伺服速度(°/s)"(1.0 ("旋转齿条轴速度(°/s)")) -> ()
            n176 = Wait (ms)(milliseconds to wait=u32 1000 ("毫秒倍数")) -> ()  [unwired: 1 out]
          }
          frame #12 {
            n177 = while {
              i -> [w262]
              stop <- w259 stop-if-true
              n178 = local read "间隙位移(mm)"() -> (w263:dbl)
              n179 = Wait Until Next ms Multiple(millisecond multiple=u32 50 ("毫秒倍数")) -> ()  [unwired: 1 out]
              n180 = Greater Or Equal?(x=w262, y=40) -> (x >= y?=w259:bool)
              n181 = local write "基准位移"(w263) -> ()
            }
          }
          frame #13 {
            n182 = call "PCI1220U运行.vi"("方向"=enum32{"Negative", "Positive"}."Negative" ("Direction"), "AxisHandle IN"=w265) -> ("AxisHandle OUT"=w264:u32)  [unwired: 9 in]
          }
          frame #14 {
            w270 = dbl[] []
            n183 = while {
              shift-right: [w281] -> w269
              shift-left: w270 -> [w283]
              shift-right: [w280] -> w268
              shift-left: w270 -> [w282]
              stop <- w273 stop-if-true
              n184 = Wait (ms)(milliseconds to wait=u32 10 ("毫秒倍数")) -> ()  [unwired: 1 out]
              n185 = local read "间隙位移(mm)"() -> (w276:dbl)
              n186 = local read "基准位移"() -> (w274:dbl)
              n187 = local read "齿条扭矩(Nm)"() -> (w277:dbl)
              n188 = Subtract(x=w276, y=w274) -> (x-y=w275:dbl)
              n189 = Absolute Value(x=w277) -> (abs(x)=w272:dbl)
              n190 = Build Array (concatenate) "创建数组"(w282, w275) -> (w280:dbl[])
              n191 = Build Array (concatenate) ("创建数组")(w283, w272) -> (w281:dbl[])
              n192 = Greater Or Equal?(x=w272, y="扭矩停止值") -> (x >= y?=w273:bool)
              n193 = Bundle ("捆绑")(w281, w280) -> (w278:cluster{dbl[], dbl[]})  [unwired: 1 in]
              n194 = Build Array ("创建数组")(w278) -> (w279:cluster{dbl[], dbl[]}[])
              n195 = local write "扭动曲线"(w279) -> ()
            }
          }
          frame #15 {
            n196 = Absolute Value(x=w293) -> (abs(x)=w294:dbl[])
            n197 = local read "测量点扭矩"() -> (w295:dbl)
            n198 = local read "基准位移"() -> (w289:dbl)
            n199 = call "自定义插值.vi"("压力"=w295, "扭矩数组"=w294, "位移数组"=w292) -> ("扭矩值"=w290:dbl)  [unwired: 8 in]
            n200 = Array Max & Min(array=w292) -> (min value=w291:dbl)  [unwired: 3 out]
            n201 = Absolute Value(x=w291) -> (abs(x)=w288:dbl)
            n202 = Subtract(x=w289, y=w288) -> (x-y=w287:dbl)
            n203 = Add(x=w290, y=w288) -> (x+y=w286:dbl)
            n204 = Absolute Value(x=w286) -> (abs(x)=w285:dbl)
            n205 = local write "基准位移"(w287) -> ()
            n206 = local write "中间位置间隙"(w285) -> ()
          }
          frame #16 {
            n207 = while {
              tunnel: w300 -> [w304]
              tunnel: [w303] -> w299
              stop <- w302 stop-if-true
              n208 = call "PCI1220U停止.vi"("AxisHandle IN"=w304) -> ("完成"=w302:bool, "AxisHandle OUT"=w303:u32)  [unwired: 9 in]
              n209 = Wait (ms)(milliseconds to wait=u32 50 ("毫秒倍数")) -> ()  [unwired: 1 out]
            }
            "间隙Y数组" <- w298
            "间隙X数组" <- w297
          }
          frame #17 {
            n210 = while {
              tunnel: [w311] -> w305
              tunnel: w306 -> [w308]
              stop <- w310 stop-if-true
              n211 = Wait Until Next ms Multiple(millisecond multiple=u32 50 ("毫秒倍数")) -> ()  [unwired: 1 out]
              n212 = call "PCI1220U扭矩轴位置模式.vi"("Distance"=0.0, "AxisHandle IN"=w308) -> ("AbsSuccess"=w310:bool, "AxisHandle OUT"=w311:u32)  [unwired: 8 in]
            }
          }
          frame #18 {
            n213 = while {
              tunnel: w313 -> [w315]
              tunnel: [w315] -> w312
              stop <- w318 stop-if-true
              n214 = local read "齿条扭矩(Nm)"() -> (w314:dbl)
              n215 = call <userlib>:"Acm_AxGetCmdVelocity.vi"("AxisHandle"=w315) -> ("Velocity"=w321:dbl)  [unwired: 1 in, 3 out]
              n216 = Wait Until Next ms Multiple(millisecond multiple=u32 50 ("毫秒倍数")) -> ()  [unwired: 1 out]
              n217 = Equal To 0?(x=w321) -> (x = 0?=w319:bool)
              n218 = Greater Or Equal?(x=w314, y=3.0) -> (x >= y?=w316:bool)
              n219 = Or(x=w319, y=w316) -> (x .or. y?=w318:bool)
            }
          }
          frame #19 {
            n220 = while {
              tunnel: w322 -> [w326]
              tunnel: [w325] -> _
              stop <- w324 stop-if-true
              n221 = call "PCI1220U停止.vi"("AxisHandle IN"=w326) -> ("完成"=w324:bool, "AxisHandle OUT"=w325:u32)  [unwired: 9 in]
              n222 = Wait (ms)(milliseconds to wait=u32 50 ("毫秒倍数")) -> ()  [unwired: 1 out]
            }
          }
          frame #20 {
            n223 = local write "旋转齿条轴使能"(FALSE ("旋转齿条轴使能")) -> ()
            n224 = Wait (ms)(milliseconds to wait=u32 500 ("毫秒倍数")) -> ()  [unwired: 1 out]
          }
          frame #21 {
            n225 = local write "工步号"(u32 25 ("工步号")) -> ()
          }
        }
      }
      frame 25 {
        n226 = flat-sequence {
          frame #0 {
            n227 = local read "中间间隙标准(mm)"() -> (w331:dbl)
            n228 = local read "最小间隙(mm)"() -> (w330:dbl)
            n229 = local read "中间位置间隙"() -> (w332:dbl)
            n230 = In Range and Coerce(upper limit=w331, x=w332, lower limit=w330) -> (In Range?=w335:bool)  [unwired: 1 out]
            n231 = case shown="假" w335 {
              tunnel: [FALSE ("本序合格") TRUE ("本序合格")] -> w334
              tunnel: [w340 0.0 ("需调整角度(度)")] -> w333
              tunnel: w332 -> [w338 _]
              tunnel: w331 -> [w337 _]
              tunnel: w330 -> [w336 _]
              frame False {
                n232 = xnode "公式"("X"=w338, "Xmax"=w337, "Xmin"=w336) -> ("结果"=w340:dbl)  [unwired: 1 in, 1 out]
              }
              frame True {
              }
            }
            n233 = local write "单点间隙合格"(w334) -> ()
            n234 = local write "需调整角度(度)"(w333) -> ()
          }
          frame #1 {
            n235 = local read "单点间隙合格"() -> (w355:bool)
            n236 = case shown="假" w355 {
              frame False {
                n237 = local read "已调试次数"() -> (w358:dbl)
                n238 = Less?(x=w358, y="设定间隙调整次数") -> (x < y?=w357:bool)
                n239 = case shown="真" w357 {
                  frame False {
                    n240 = local write "工步号"(u32 45 ("变更工步号")) -> ()
                  }
                  frame True {
                    n241 = local write "工步号"(u32 30 ("变更工步号")) -> ()
                  }
                }
              }
              frame True {
                n242 = local write "工步号"(u32 40 ("变更工步号")) -> ()
              }
            }
          }
        }
      }
      frame 30 {
        # "人工调整"
        n243 = flat-sequence {
          tunnel: [w364] -> w362
          tunnel: w362 -> [w371]
          frame #0 {
            n244 = local write "测头机构轴速度(mm/s)"(30.0 ("测头机构轴速度(mm/s)")) -> ()
          }
          frame #1 {
            n245 = local read "测头机构电机"() -> (w365:u32)
            n246 = while {
              tunnel: w365 -> [w368]
              tunnel: [w367] -> w364
              stop <- w370 stop-if-true
              n247 = local read "测头机构轴待检位"() -> (w366:dbl)
              n248 = call "PCI1220U进给轴位置模式.vi"("Distance"=w366, "AxisHandle IN"=w368) -> ("AbsSuccess"=w370:bool, "AxisHandle OUT"=w367:u32)  [unwired: 8 in]
              n249 = Wait Until Next ms Multiple(millisecond multiple=u32 50 ("毫秒倍数")) -> ()  [unwired: 1 out]
            }
          }
          frame #2 {
            n250 = while {
              tunnel: w371 -> [w375]
              stop <- w373 stop-if-true
              n251 = call <userlib>:"Acm_AxGetCmdVelocity.vi"("AxisHandle"=w375) -> ("Velocity"=w374:dbl)  [unwired: 1 in, 3 out]
              n252 = Wait Until Next ms Multiple(millisecond multiple=u32 50 ("毫秒倍数")) -> ()  [unwired: 1 out]
              n253 = Equal To 0?(x=w374) -> (x = 0?=w373:bool)
            }
          }
          frame #3 {
            n254 = while {
              stop <- w377 stop-if-true
              n255 = local read "测头机构轴位置(mm)"() -> (w379:dbl)
              n256 = Wait Until Next ms Multiple(millisecond multiple=u32 50 ("毫秒倍数")) -> ()  [unwired: 1 out]
              n257 = Less Or Equal?(x=w379, y=35.0) -> (x <= y?=w377:bool)
            }
          }
          frame #4 {
            n258 = local write "测头气缸左移"(TRUE ("测头气缸左移")) -> ()
            n259 = local write "测头气缸右移"(FALSE ("测头气缸右移")) -> ()
          }
          frame #5 {
            n260 = while {
              stop <- w382 stop-if-true
              # "等待启动"
              n261 = local read "间隙启动"() -> (w382:bool)
              n262 = Wait Until Next ms Multiple(millisecond multiple=u32 50 ("毫秒倍数")) -> ()  [unwired: 1 out]
            }
          }
          frame #6 {
            n263 = local read "不合格品"() -> (w384:bool)
            n264 = case shown="假" w384 {
              frame False {
                n265 = flat-sequence {
                  frame #0 {
                    n266 = local read "已调试次数"() -> (w387:dbl)
                    n267 = local write "测头气缸左移"(FALSE ("测头气缸左移")) -> ()
                    n268 = local write "测头气缸右移"(TRUE ("测头气缸左移")) -> ()
                    n269 = Add(x=w387, y=1.0 ("已调试次数")) -> (x+y=w389:dbl)
                    n270 = local write "已调试次数"(w389) -> ()
                  }
                  frame #1 {
                    n271 = while {
                      stop <- w390 stop-if-true
                      n272 = Wait Until Next ms Multiple(millisecond multiple=u32 50 ("毫秒倍数")) -> ()  [unwired: 1 out]
                      n273 = local read "测头右位"() -> (w390:bool)
                    }
                  }
                  frame #2 {
                    n274 = local write "工步号"(u32 20 ("工步号")) -> ()
                  }
                }
              }
              frame True {
                n275 = local write "工步号"(u32 45 ("工步号")) -> ()
              }
            }
          }
        }
      }
      frame 40 {
        n276 = flat-sequence {
          tunnel: [w492] -> w488
          tunnel: w488 -> [w494]
          tunnel: [w493] -> w486
          tunnel: w486 -> [w500]
          tunnel: [w500] -> w471
          tunnel: w471 -> [w509]
          tunnel: [w509] -> w470
          tunnel: w470 -> [w516]
          tunnel: [w516] -> w485
          tunnel: w485 -> [w518]
          tunnel: [w519] -> w469
          tunnel: [w517] -> w468
          tunnel: [w531] -> w478
          tunnel: [w530] -> w477
          tunnel: [w529] -> w476
          tunnel: w469 -> [w528]
          tunnel: [w528] -> w475
          tunnel: [w526] -> w473
          tunnel: w468 -> [w525]
          tunnel: w478 -> [w571]
          tunnel: [w571] -> w445
          tunnel: w477 -> [w578]
          tunnel: [w578] -> w443
          tunnel: w476 -> [w574]
          tunnel: [w574] -> w441
          tunnel: w475 -> [w577]
          tunnel: [w577] -> w439
          tunnel: [w573] -> w437
          tunnel: w473 -> [w573]
          tunnel: [w575] -> w435
          tunnel: [w565] -> w433
          tunnel: [w572] -> w431
          tunnel: [w566] -> w429
          tunnel: [w570] -> w427
          tunnel: [w569] -> w425
          tunnel: [w567] -> w424
          tunnel: [w568] -> w423
          tunnel: [w564] -> w398
          tunnel: w445 -> [w598]
          tunnel: [w598] -> w444
          tunnel: w443 -> [w597]
          tunnel: [w597] -> w442
          tunnel: w441 -> [w596]
          tunnel: [w596] -> w440
          tunnel: w439 -> [w595]
          tunnel: [w595] -> w438
          tunnel: w437 -> [w594]
          tunnel: [w594] -> w436
          tunnel: w435 -> [w593]
          tunnel: [w593] -> w434
          tunnel: w433 -> [w592]
          tunnel: [w592] -> w432
          tunnel: w431 -> [w591]
          tunnel: [w591] -> w430
          tunnel: w429 -> [w590]
          tunnel: [w590] -> w428
          tunnel: w427 -> [w589]
          tunnel: [w589] -> w426
          tunnel: w425 -> [w584]
          tunnel: w424 -> [w586]
          tunnel: w423 -> [w585]
          tunnel: w398 -> [w583]
          tunnel: w444 -> [w615]
          tunnel: [w615] -> w484
          tunnel: w442 -> [w614]
          tunnel: [w614] -> w483
          tunnel: w440 -> [w613]
          tunnel: [w613] -> w482
          tunnel: w438 -> [w612]
          tunnel: [w612] -> w480
          tunnel: [w611] -> w474
          tunnel: w436 -> [w611]
          tunnel: [w610] -> w472
          tunnel: w434 -> [w610]
          tunnel: w432 -> [w606]
          tunnel: w430 -> [w609]
          tunnel: w428 -> [w607]
          tunnel: w426 -> [w608]
          tunnel: [w608] -> w449
          tunnel: [w600] -> w413
          tunnel: [w599] -> w412
          tunnel: [w632] -> w467
          tunnel: [w631] -> w466
          tunnel: w484 -> [w620]
          tunnel: w483 -> [w630]
          tunnel: w482 -> [w629]
          tunnel: [w628] -> w464
          tunnel: w480 -> [w627]
          tunnel: [w627] -> w462
          tunnel: w474 -> [w626]
          tunnel: w472 -> [w624]
          tunnel: [w625] -> w460
          tunnel: [w624] -> w458
          tunnel: w449 -> [w623]
          tunnel: [w623] -> w448
          tunnel: w413 -> [w622]
          tunnel: w412 -> [w621]
          tunnel: [w622] -> w411
          tunnel: [w621] -> w410
          tunnel: w467 -> [w668]
          tunnel: w466 -> [w677]
          tunnel: [w677] -> w465
          tunnel: w464 -> [w673]
          tunnel: [w673] -> w463
          tunnel: w462 -> [w676]
          tunnel: [w676] -> w461
          tunnel: w460 -> [w675]
          tunnel: [w675] -> w459
          tunnel: w458 -> [w674]
          tunnel: [w674] -> w457
          tunnel: [w670] -> w451
          tunnel: [w669] -> w450
          tunnel: w448 -> [w667]
          tunnel: [w668] -> w447
          tunnel: [w667] -> w446
          tunnel: w411 -> [w666]
          tunnel: w410 -> [w665]
          tunnel: [w666] -> w406
          tunnel: [w665] -> w403
          tunnel: w465 -> [w711]
          tunnel: [w723] -> w487
          tunnel: w463 -> [w723]
          tunnel: [w722] -> w479
          tunnel: w461 -> [w722]
          tunnel: w459 -> [w721]
          tunnel: w457 -> [w720]
          tunnel: [w718] -> w456
          tunnel: w451 -> [w717]
          tunnel: w450 -> [w716]
          tunnel: w447 -> [w699]
          tunnel: w446 -> [w698]
          tunnel: [w707] -> w422
          tunnel: [w706] -> w409
          tunnel: [w705] -> w407
          tunnel: w406 -> [w705]
          tunnel: [w704] -> w404
          tunnel: w403 -> [w704]
          tunnel: [w703] -> w401
          tunnel: [w702] -> w399
          tunnel: [w685] -> w396
          tunnel: [w686] -> w394
          tunnel: w487 -> [w744]
          tunnel: [w744] -> w421
          tunnel: w479 -> [_]
          tunnel: [w740] -> w419
          tunnel: w456 -> [w742]
          tunnel: [w739] -> w417
          tunnel: w422 -> [w738]
          tunnel: [w726] -> w415
          tunnel: [w736] -> w414
          tunnel: w409 -> [w735]
          tunnel: [w730] -> w408
          tunnel: w407 -> [w730]
          tunnel: [w729] -> w405
          tunnel: w404 -> [w729]
          tunnel: [w728] -> w402
          tunnel: w401 -> [w728]
          tunnel: [w727] -> w400
          tunnel: w399 -> [w727]
          tunnel: [w725] -> w397
          tunnel: w396 -> [w725]
          tunnel: [w724] -> w395
          tunnel: w394 -> [w724]
          tunnel: w421 -> [w757]
          tunnel: [w757] -> w420
          tunnel: w419 -> [w756]
          tunnel: [w756] -> w418
          tunnel: w417 -> [w755]
          tunnel: [w755] -> w416
          tunnel: w415 -> [w751]
          tunnel: w414 -> [w747]
          tunnel: w408 -> [w750]
          tunnel: w405 -> [w749]
          tunnel: w402 -> [w753]
          tunnel: w400 -> [w752]
          tunnel: w397 -> [w746]
          tunnel: w395 -> [w745]
          tunnel: w420 -> [w761]
          tunnel: [w760] -> w481
          tunnel: w418 -> [w759]
          tunnel: [w758] -> w452
          tunnel: w416 -> [w758]
          tunnel: w481 -> [w768]
          tunnel: [w768] -> w455
          tunnel: [w767] -> w453
          tunnel: w452 -> [w767]
          tunnel: w455 -> [w775]
          tunnel: [w774] -> w454
          tunnel: w453 -> [w773]
          tunnel: w454 -> [w781]
          frame #0 {
            n277 = local write "电动缸速度(mm/s)"(15.0 ("电动缸速度(mm/s)")) -> ()
            n278 = local write "已调试次数"(0.0 ("已调试次数")) -> ()
            n279 = local write "选项卡控件"(T1."轴向力测量" ("选项卡控件")) -> ()
            n280 = local read "电动缸电机"() -> (w492:u32)
          }
          frame #1 {
            n281 = while {
              tunnel: w494 -> [w499]
              tunnel: [w498] -> w493
              stop <- w497 stop-if-true
              n282 = local read "齿条左极限"() -> (w495:dbl)
              n283 = Wait (ms)(milliseconds to wait=u32 50 ("毫秒倍数")) -> ()  [unwired: 1 out]
              n284 = call "PCI1240电动缸位置模式 .vi"("Distance"=w495, "AxisHandle IN"=w499) -> ("AbsSuccess"=w497:bool, "AxisHandle OUT"=w498:u32)  [unwired: 8 in]
            }
          }
          frame #2 {
            n285 = while {
              tunnel: w500 -> [w508]
              stop <- w501 stop-if-true
              n286 = local read "齿条推拉力(N)"() -> (w505:dbl)
              n287 = call <userlib>:"Acm_AxGetCmdVelocity.vi"("AxisHandle"=w508) -> ("Velocity"=w507:dbl)  [unwired: 1 in, 3 out]
              n288 = Wait Until Next ms Multiple(millisecond multiple=u32 50 ("毫秒倍数")) -> ()  [unwired: 1 out]
              n289 = Equal To 0?(x=w507) -> (x = 0?=w503:bool)
              n290 = Less Or Equal?(x=w505, y=-1000.0) -> (x <= y?=w502:bool)
              n291 = Or ("或")(x=w503, y=w502) -> (x .or. y?=w501:bool)
            }
          }
          frame #3 {
            n292 = while {
              tunnel: w509 -> [w513]
              tunnel: [w512] -> _
              stop <- w511 stop-if-true
              n293 = call "PCI1220U停止.vi"("AxisHandle IN"=w513) -> ("完成"=w511:bool, "AxisHandle OUT"=w512:u32)  [unwired: 9 in]
              n294 = Wait (ms)(milliseconds to wait=u32 50 ("毫秒倍数")) -> ()  [unwired: 1 out]
            }
          }
          frame #4 {
            n295 = Wait Until Next ms Multiple(millisecond multiple=u32 50 ("毫秒倍数")) -> ()  [unwired: 1 out]
            n296 = local write "电动缸速度(mm/s)"(15.0 ("电动缸速度(mm/s)")) -> ()
          }
          frame #5 {
            n297 = while {
              tunnel: w518 -> [w524]
              tunnel: [w521] -> w517
              stop <- w522 stop-if-true
              n298 = local read "齿条右极限"() -> (w520:dbl)
              n299 = Wait Until Next ms Multiple(millisecond multiple=u32 50 ("毫秒倍数")) -> ()  [unwired: 1 out]
              n300 = call "PCI1240电动缸位置模式 .vi"("Distance"=w520, "AxisHandle IN"=w524) -> ("AbsSuccess"=w522:bool, "AxisHandle OUT"=w521:u32)  [unwired: 8 in]
            }
            n301 = local read "转向器中心"() -> (w519:dbl)
          }
          frame #6 {
            w527 = dbl[] []
            n302 = while {
              shift-right: [w552] -> w530
              shift-left: w527 -> [w562]
              shift-right: [w560] -> w531
              shift-left: w527 -> [w561]
              tunnel: w525 -> [w557]
              tunnel: [w557] -> w529
              tunnel: w528 -> [w555]
              shift-right: [w551] -> w526
              shift-left: w527 -> [w553]
              stop <- w545 stop-if-true
              n303 = local read "中间位置间隙"() -> (w542:dbl)
              n304 = local read "基准位移"() -> (w558:dbl)
              n305 = local read "间隙位移(mm)"() -> (w541:dbl)
              n306 = call <userlib>:"Acm_AxGetCmdVelocity.vi"("AxisHandle"=w557) -> ("Velocity"=w550:dbl)  [unwired: 1 in, 3 out]
              n307 = Wait (ms)(milliseconds to wait=u32 50 ("毫秒倍数")) -> ()  [unwired: 1 out]
              n308 = local read "齿条推拉力(N)"() -> (w548:dbl)
              n309 = call "PCI1240电动缸读取位置.vi"("AxisHandle IN"=w557) -> ("位置"=w556:dbl)  [unwired: 9 in, 1 out]
              n310 = Subtract(x=w541, y=w558) -> (x-y=w544:dbl)
              n311 = Subtract(x=w556, y=w555) -> (x-y=w535:dbl)
              n312 = Add(x=w544, y=w542) -> (x+y=w543:dbl)
              n313 = Multiply(x=w535, y=1.12) -> (x*y=w533:dbl)
              n314 = Build Array (concatenate) ("创建数组")(w561, w543) -> (w560:dbl[])
              n315 = Build Array (concatenate) ("创建数组")(w562, w533) -> (w552:dbl[])
              n316 = Build Array (concatenate) ("创建数组")(w553, w548) -> (w551:dbl[])
              n317 = Greater Or Equal?(x=w548, y=1000.0) -> (x >= y?=w546:bool)
              n318 = Less Or Equal?(x=w541, y=0.0) -> (x <= y?=w540:bool)
              n319 = Greater Or Equal?(x=w541, y=4.0) -> (x >= y?=w539:bool)
              n320 = Equal To 0?(x=w550) -> (x = 0?=w547:bool)
              n321 = Or(x=w539, y=w540) -> (x .or. y?=w538:bool)
              n322 = Bundle ("捆绑")(w552, w560) -> (w532:cluster{dbl[], dbl[]})  [unwired: 1 in]
              n323 = Or(x=w547, y=w546) -> (x .or. y?=w545:bool)
              n324 = Bundle ("捆绑")(w552, w551) -> (w554:cluster{dbl[], dbl[]})  [unwired: 1 in]
              n325 = property on="间隙位移(mm)" class="DigNum (严格)"("Blinking"=w538) -> ()  [unwired: 2 in, 2 out]
              n326 = Build Array ("创建数组")(w532, w554) -> (w559:cluster{dbl[], dbl[]}[])
              n327 = local write "行程跳动曲线"(w559) -> ()
            }
          }
          frame #7 {
            n328 = Wait Until Next ms Multiple(millisecond multiple=u32 500 ("毫秒倍数")) -> ()  [unwired: 1 out]
            n329 = while {
              tunnel: w574 -> [w582]
              tunnel: [w581] -> _
              stop <- w580 stop-if-true
              n330 = call "PCI1220U停止.vi"("AxisHandle IN"=w582) -> ("完成"=w580:bool, "AxisHandle OUT"=w581:u32)  [unwired: 9 in]
              n331 = Wait (ms)(milliseconds to wait=u32 50 ("毫秒倍数")) -> ()  [unwired: 1 out]
            }
            n332 = Array Size(array=w573) -> (size(s)=w575:i32)
            n333 = call "间隙计算.vi"("扭矩数组"=w571) -> ("峰值间隙1"=w567:dbl, "峰值间隙2"=w568:dbl)  [unwired: 6 in, 3 out]
            n334 = call "功能计算.vi"("扭矩数组"=w573) -> ("扭差"=w566:dbl, "平均扭矩"=w572:dbl, "峰值扭矩"=w565:dbl)  [unwired: 7 in, 1 out]
            n335 = Array Size(array=w571) -> (size(s)=w570:i32)
            n336 = local read "全行程180°外间隙标准(mm)"() -> (w564:dbl)
            n337 = local read "全行程180°内间隙标准(mm)"() -> (w569:dbl)
            n338 = local write "左180°内全行程间隙"(w567) -> ()
            n339 = local write "左180°外全行程间隙"(w568) -> ()
            n340 = local write "左最大轴向力(N)"(w565) -> ()
            n341 = local write "左平均轴向力(N)"(w572) -> ()
            n342 = local write "左轴向力波动(N)"(w566) -> ()
          }
          frame #8 {
            n343 = Greater?(x=w585, y=w583) -> (0:w587:bool)
            n344 = Greater?(x=w586, y=w584) -> (0:w588:bool)
            n345 = property on="左180°外全行程间隙" class="DigNum (严格)"("Blinking"=w587) -> ()  [unwired: 2 in, 2 out]
            n346 = property on="左180°内全行程间隙" class="DigNum (严格)"("Blinking"=w588) -> ()  [unwired: 2 in, 2 out]
          }
          frame #9 {
            n347 = local read "最大轴向力标准(N)"() -> (w604:dbl)
            n348 = while {
              tunnel: w613 -> [w619]
              tunnel: w612 -> [_]
              stop <- w618 stop-if-true
              n349 = local read "齿条左极限"() -> (w616:dbl)
              n350 = Wait Until Next ms Multiple(millisecond multiple=u32 50 ("毫秒倍数")) -> ()  [unwired: 1 out]
              n351 = call "PCI1240电动缸位置模式 .vi"("Distance"=w616, "AxisHandle IN"=w619) -> ("AbsSuccess"=w618:bool)  [unwired: 8 in, 1 out]
            }
            n352 = local read "轴向力标准(N)"() -> (w603:dbl)
            n353 = local read "平均轴向力MAX(N)"() -> (w602:dbl)
            n354 = local read "力波动标准(N)"() -> (w601:dbl)
            n355 = call "判断.vi"("y 3"=w601, "y2-2"=w602, "y2-1"=w603, "y"=w604, "x 3"=w607, "x 2"=w609, "x"=w606) -> ("非x? 3"=w599:bool, "非x? 2"=w605:bool, "非x?"=w600:bool)  [unwired: 2 in]
            n356 = property on="左最大轴向力(N)" class="DigNum (严格)"("Blinking"=w600) -> ()  [unwired: 2 in, 2 out]
            n357 = property on="左轴向力波动(N)" class="DigNum (严格)"("Blinking"=w599) -> ()  [unwired: 2 in, 2 out]
            n358 = property on="左平均轴向力(N)" class="DigNum (严格)"("Blinking"=w605) -> ()  [unwired: 2 in, 2 out]
          }
          frame #10 {
            n359 = while {
              shift-right: [w634] -> w631
              shift-left: w630 -> [w663]
              shift-right: [w661] -> w632
              shift-left: w620 -> [w662]
              tunnel: w629 -> [w658]
              tunnel: [w658] -> w628
              tunnel: w627 -> [w656]
              shift-right: [w653] -> w625
              shift-left: w626 -> [w654]
              stop <- w648 stop-if-true
              n360 = local read "间隙位移(mm)"() -> (w640:dbl)
              n361 = call <userlib>:"Acm_AxGetCmdVelocity.vi"("AxisHandle"=w658) -> ("Velocity"=w646:dbl)  [unwired: 1 in, 3 out]
              n362 = local read "基准位移"() -> (w659:dbl)
              n363 = Wait (ms)(milliseconds to wait=u32 50 ("毫秒倍数")) -> ()  [unwired: 1 out]
              n364 = local read "中间位置间隙"() -> (w645:dbl)
              n365 = local read "齿条推拉力(N)"() -> (w652:dbl)
              n366 = call "PCI1240电动缸读取位置.vi"("AxisHandle IN"=w658) -> ("位置"=w657:dbl)  [unwired: 9 in, 1 out]
              n367 = Subtract(x=w640, y=w659) -> (x-y=w660:dbl)
              n368 = Subtract(x=w657, y=w656) -> (x-y=w638:dbl)
              n369 = Add(x=w660, y=w645) -> (x+y=w647:dbl)
              n370 = Multiply(x=w638, y=1.12) -> (x*y=w636:dbl)
              n371 = Less Or Equal?(x=w652, y=-1000.0) -> (x <= y?=w649:bool)
              n372 = Build Array (concatenate) ("创建数组")(w663, w636) -> (w634:dbl[])
              n373 = Build Array (concatenate) ("创建数组")(w654, w652) -> (w653:dbl[])
              n374 = Equal To 0?(x=w646) -> (x = 0?=w650:bool)
              n375 = Build Array (concatenate) ("创建数组")(w662, w647) -> (w661:dbl[])
              n376 = Bundle ("捆绑")(w634, w653) -> (w655:cluster{dbl[], dbl[]})  [unwired: 1 in]
              n377 = Or(x=w650, y=w649) -> (x .or. y?=w648:bool)
              n378 = Bundle ("捆绑")(w634, w661) -> (w635:cluster{dbl[], dbl[]})  [unwired: 1 in]
              n379 = Build Array ("创建数组")(w635, w655) -> (w633:cluster{dbl[], dbl[]}[])
              n380 = Less Or Equal?(x=w640, y=0.0) -> (x <= y?=w644:bool)
              n381 = Greater Or Equal?(x=w640, y=4.0) -> (x >= y?=w643:bool)
              n382 = Or(x=w643, y=w644) -> (x .or. y?=w639:bool)
              n383 = local write "行程跳动曲线"(w633) -> ()
              n384 = property on="间隙位移(mm)" class="DigNum (严格)"("Blinking"=w639) -> ()  [unwired: 2 in, 2 out]
            }
          }
          frame #11 {
            n385 = while {
              tunnel: w673 -> [w681]
              tunnel: [w680] -> _
              stop <- w679 stop-if-true
              n386 = call "PCI1220U停止.vi"("AxisHandle IN"=w681) -> ("完成"=w679:bool, "AxisHandle OUT"=w680:u32)  [unwired: 9 in]
              n387 = Wait (ms)(milliseconds to wait=u32 50 ("毫秒倍数")) -> ()  [unwired: 1 out]
            }
            n388 = Array Max & Min(array=w668) -> (max value=w672:dbl, min value=w671:dbl)  [unwired: 2 out]
            n389 = Absolute Value(x=w672) -> (abs(x)=w670:dbl)
            n390 = Absolute Value(x=w671) -> (abs(x)=w669:dbl)
            n391 = local write "右全行程间隙"(w669) -> ()
            n392 = local write "左全行程间隙"(w670) -> ()
          }
          frame #12 {
            n393 = local read "全行程180°外间隙标准(mm)"() -> (w715:dbl)
            n394 = local read "全行程180°外间隙标准(mm)"() -> (w695:dbl)
            n395 = Split 1D Array(array=w721, index=w720) -> (second subarray=w719:dbl[])  [unwired: 1 out]
            n396 = local read "全行程180°内间隙标准(mm)"() -> (w696:dbl)
            n397 = Array Max & Min(array=w711) -> (max value=w710:dbl, min value=w709:dbl)  [unwired: 2 out]
            n398 = local read "总行程标准(mm)"() -> (w690:dbl)
            n399 = call "功能计算.vi"("扭矩数组"=w719) -> ("扭差"=w706:dbl, "平均扭矩"=w718:dbl, "峰值扭矩"=w707:dbl)  [unwired: 7 in, 1 out]
            n400 = Split 1D Array(array=w699, index=w698) -> (second subarray=w697:dbl[])  [unwired: 1 out]
            n401 = Subtract(x=w710, y=w709) -> (x-y=w701:dbl)
            n402 = Subtract(x=w701, y="全行程修正") -> (x-y=w683:dbl)
            n403 = Subtract(x=w683, y="机械间隙值") -> (x-y=w682:dbl)
            n404 = local write "总行程(mm)"(w682) -> ()
            n405 = local write "右最大轴向力(N)"(w707) -> ()
            n406 = Greater?(x=w717, y=w715) -> (0:w703:bool)
            n407 = call "间隙计算.vi"("扭矩数组"=w697) -> ("峰值间隙1"=w714:dbl, "峰值间隙2"=w713:dbl)  [unwired: 6 in, 3 out]
            n408 = Greater?(x=w716, y=w715) -> (0:w702:bool)
            n409 = local write "右轴向力波动(N)"(w706) -> ()
            n410 = local read "总行程最大值"() -> (w691:dbl)
            n411 = In Range and Coerce "判定范围并强制转换"(upper limit=w691, x=w682, lower limit=w690) -> (In Range?=w688:bool)  [unwired: 1 out]
            n412 = Greater?(x=w713, y=w695) -> (0:w689:bool)
            n413 = Greater?(x=w714, y=w696) -> (0:w712:bool)
            n414 = local write "右平均轴向力(N)"(w718) -> ()
            n415 = local write "右180°外全行程间隙"(w713) -> ()
            n416 = local read "总圈数最大值"() -> (w692:dbl)
            n417 = local write "右180°内全行程间隙"(w714) -> ()
            n418 = property on="左全行程间隙" class="DigNum (严格)"("Blinking"=w703) -> ()  [unwired: 2 in, 2 out]
            n419 = property on="右全行程间隙" class="DigNum (严格)"("Blinking"=w702) -> ()  [unwired: 2 in, 2 out]
            n420 = Divide(x=w682, y=46.996) -> (x/y=w694:dbl)
            n421 = property on="右180°外全行程间隙" class="DigNum (严格)"("Blinking"=w689) -> ()  [unwired: 2 in, 2 out]
            n422 = local read "总圈数标准"() -> (w693:dbl)
            n423 = In Range and Coerce(upper limit=w692, x=w694, lower limit=w693) -> (In Range?=w687:bool)  [unwired: 1 out]
            n424 = Not(x=w688) -> (.not. x?=w686:bool)
            n425 = local write "总圈数"(w694) -> ()
            n426 = Not(x=w687) -> (.not. x?=w685:bool)
            n427 = property on="右180°内全行程间隙" class="DigNum (严格)"("Blinking"=w712) -> ()  [unwired: 2 in, 2 out]
            n428 = property on="总行程(mm)" class="DigNum (严格)"("Blinking"=w686) -> ()  [unwired: 2 in, 2 out]
            n429 = property on="总圈数" class="DigNum (严格)"("Blinking"=w685) -> ()  [unwired: 2 in, 2 out]
            "轴向力X" <- w711
            "轴向力Y" <- w721
          }
          frame #13 {
            n430 = local read "最大轴向力标准(N)"() -> (w734:dbl)
            n431 = local read "转向器中心"() -> (w739:dbl)
            n432 = local read "平均轴向力MAX(N)"() -> (w732:dbl)
            n433 = local read "轴向力标准(N)"() -> (w733:dbl)
            n434 = local read "力波动标准(N)"() -> (w731:dbl)
            n435 = call "判断.vi"("y 3"=w731, "y2-2"=w732, "y2-1"=w733, "y"=w734, "x 3"=w735, "x 2"=w742, "x"=w738) -> ("非x? 3"=w736:bool, "非x? 2"=w737:bool, "非x?"=w726:bool)  [unwired: 2 in]
            n436 = local write "电动缸速度(mm/s)"(15.0 ("电动缸速度(mm/s)")) -> ()
            n437 = property on="右最大轴向力(N)" class="DigNum (严格)"("Blinking"=w726) -> ()  [unwired: 2 in, 2 out]
            n438 = property on="右平均轴向力(N)" class="DigNum (严格)"("Blinking"=w737) -> ()  [unwired: 2 in, 2 out]
            n439 = Add(x=w739, y=-10.0) -> (x+y=w740:dbl)
          }
          frame #14 {
            n440 = Compound Arithmetic op=OR(w746, w753, w752, w751, w747, w750, w749, w745) -> (w748:bool)
            n441 = property on="右轴向力波动(N)" class="DigNum (严格)"("Blinking"=w747) -> ()  [unwired: 2 in, 2 out]
            n442 = Not(x=w748) -> (.not. x?=w754:bool)
            n443 = local write "全行程间隙及轴向力合格"(w754) -> ()
          }
          frame #15 {
            n444 = while {
              tunnel: w761 -> [w765]
              tunnel: [w763] -> w760
              tunnel: w759 -> [w762]
              stop <- w764 stop-if-true
              n445 = call "PCI1240电动缸位置模式 .vi"("Distance"=w762, "AxisHandle IN"=w765) -> ("AbsSuccess"=w764:bool, "AxisHandle OUT"=w763:u32)  [unwired: 8 in]
              n446 = Wait (ms)(milliseconds to wait=u32 50 ("毫秒倍数")) -> ()  [unwired: 1 out]
            }
          }
          frame #16 {
            n447 = while {
              tunnel: w768 -> [w772]
              stop <- w770 stop-if-true
              n448 = call <userlib>:"Acm_AxGetCmdVelocity.vi"("AxisHandle"=w772) -> ("Velocity"=w771:dbl)  [unwired: 1 in, 3 out]
              n449 = Wait Until Next ms Multiple(millisecond multiple=u32 50 ("毫秒倍数")) -> ()  [unwired: 1 out]
              n450 = Equal To 0?(x=w771) -> (x = 0?=w770:bool)
            }
          }
          frame #17 {
            n451 = while {
              tunnel: w775 -> [w779]
              tunnel: [w777] -> w774
              tunnel: w773 -> [w776]
              stop <- w778 stop-if-true
              n452 = call "PCI1240电动缸位置模式 .vi"("Distance"=w776, "AxisHandle IN"=w779) -> ("AbsSuccess"=w778:bool, "AxisHandle OUT"=w777:u32)  [unwired: 8 in]
              n453 = Wait (ms)(milliseconds to wait=u32 50 ("毫秒倍数")) -> ()  [unwired: 1 out]
            }
          }
          frame #18 {
            n454 = while {
              tunnel: w781 -> [w785]
              stop <- w783 stop-if-true
              n455 = call <userlib>:"Acm_AxGetCmdVelocity.vi"("AxisHandle"=w785) -> ("Velocity"=w784:dbl)  [unwired: 1 in, 3 out]
              n456 = Wait Until Next ms Multiple(millisecond multiple=u32 50 ("毫秒倍数")) -> ()  [unwired: 1 out]
              n457 = Equal To 0?(x=w784) -> (x = 0?=w783:bool)
            }
          }
          frame #19 {
            n458 = local read "轴向力已做次数"() -> (w788:dbl)
            n459 = Add(x=w788, y=1.0) -> (x+y=w786:dbl)
            n460 = local write "轴向力已做次数"(w786) -> ()
          }
          frame #20 {
            n461 = local read "全行程间隙及轴向力合格"() -> (w789:bool)
            n462 = case shown="假" w789 {
              frame False {
                n463 = Less?(x="轴向力已做次数", y="设定轴向力调整次数") -> (x < y?=w791:bool)
                n464 = case shown="真" w791 {
                  frame False {
                    n465 = local write "工步号"(u32 45 ("工步号")) -> ()
                  }
                  frame True {
                    n466 = local write "工步号"(u32 30 ("工步号")) -> ()
                  }
                }
              }
              frame True {
                n467 = local write "工步号"(u32 45 ("工步号")) -> ()
              }
            }
          }
        }
      }
      frame 45 {
        # "测头退回"
        n468 = flat-sequence {
          tunnel: [w799] -> w796
          tunnel: w796 -> [w806]
          frame #0 {
            n469 = local write "测头机构轴速度(mm/s)"(30.0 ("测头机构轴速度(mm/s)")) -> ()
          }
          frame #1 {
            n470 = local read "测头机构轴后退位"() -> (w798:dbl)
            n471 = local read "测头机构电机"() -> (w800:u32)
            n472 = while {
              tunnel: w800 -> [w804]
              tunnel: w798 -> [w803]
              tunnel: [w802] -> w799
              stop <- w805 stop-if-true
              n473 = Wait Until Next ms Multiple(millisecond multiple=u32 50 ("毫秒倍数")) -> ()  [unwired: 1 out]
              n474 = call "PCI1220U进给轴位置模式.vi"("Distance"=w803, "AxisHandle IN"=w804) -> ("AbsSuccess"=w805:bool, "AxisHandle OUT"=w802:u32)  [unwired: 8 in]
            }
          }
          frame #2 {
            n475 = while {
              tunnel: w806 -> [w810]
              stop <- w808 stop-if-true
              n476 = call <userlib>:"Acm_AxGetCmdVelocity.vi"("AxisHandle"=w810) -> ("Velocity"=w809:dbl)  [unwired: 1 in, 3 out]
              n477 = Wait Until Next ms Multiple(millisecond multiple=u32 50 ("毫秒倍数")) -> ()  [unwired: 1 out]
              n478 = Equal To 0?(x=w809) -> (x = 0?=w808:bool)
            }
          }
          frame #3 {
            n479 = while {
              stop <- w811 stop-if-true
              n480 = local read "测头机构轴位置(mm)"() -> (w813:dbl)
              n481 = Wait Until Next ms Multiple(millisecond multiple=u32 50 ("毫秒倍数")) -> ()  [unwired: 1 out]
              n482 = Less Or Equal?(x=w813, y=35.0) -> (x <= y?=w811:bool)
            }
          }
          frame #4 {
            n483 = local write "测头气缸左移"(TRUE ("测头气缸左移")) -> ()
            n484 = local write "测头气缸右移"(FALSE ("测头气缸右移")) -> ()
          }
          frame #5 {
            n485 = Wait Until Next ms Multiple(millisecond multiple=u32 500 ("毫秒倍数")) -> ()  [unwired: 1 out]
          }
          frame #6 {
            n486 = local write "工步号"(u32 50 ("工步号")) -> ()
          }
        }
      }
      frame 50 {
        n487 = flat-sequence {
          tunnel: [w840] -> w829
          tunnel: w829 -> [w847]
          tunnel: [w846] -> w827
          tunnel: w827 -> [w858]
          tunnel: [w865] -> w821
          tunnel: [w869] -> w822
          tunnel: w821 -> [w869]
          tunnel: [w872] -> w824
          tunnel: w822 -> [w871]
          tunnel: w824 -> [w879]
          tunnel: [w878] -> w823
          tunnel: w823 -> [w881]
          tunnel: [w880] -> w819
          tunnel: [w886] -> w820
          tunnel: w819 -> [w886]
          tunnel: [w889] -> w828
          tunnel: w820 -> [w888]
          tunnel: w828 -> [w895]
          tunnel: [w896] -> w826
          tunnel: w826 -> [w905]
          tunnel: [w904] -> w825
          tunnel: w825 -> [w915]
          frame #0 {
            n488 = local write "旋转伺服速度(°/s)"(15.0 ("调整螺塞轴速度(°/s)")) -> ()
            n489 = local write "测头机构轴速度(mm/s)"(15.0 ("调整机构轴速度(mm/s)")) -> ()
            n490 = local write "电动缸速度(mm/s)"(15.0 ("电动缸速度(mm/s)")) -> ()
            n491 = local write "夹头松开"(TRUE ("夹头松开")) -> ()
            n492 = local write "夹头夹紧"(FALSE ("夹头夹紧")) -> ()
          }
          frame #1 {
            n493 = while {
              stop <- w835 stop-if-true
              n494 = local read "夹头夹紧位"() -> (w838:bool)
              n495 = local read "夹头松开"() -> (w836:bool)
              n496 = Wait Until Next ms Multiple(millisecond multiple=u32 50 ("毫秒倍数")) -> ()  [unwired: 1 out]
              n497 = Not(x=w838) -> (.not. x?=w837:bool)
              n498 = And(x=w837, y=w836) -> (x .and. y?=w835:bool)
            }
          }
          frame #2 {
            n499 = while {
              tunnel: [w843] -> w840
              stop <- w842 stop-if-true
              n500 = local read "电动缸电机"() -> (w844:u32)
              n501 = Wait Until Next ms Multiple(millisecond multiple=u32 50 ("毫秒倍数")) -> ()  [unwired: 1 out]
              n502 = local read "齿条右极限"() -> (w841:dbl)
              n503 = call "PCI1240电动缸位置模式 .vi"("Distance"=w841, "AxisHandle IN"=w844) -> ("AbsSuccess"=w842:bool, "AxisHandle OUT"=w843:u32)  [unwired: 8 in]
            }
          }
          frame #3 {
            n504 = while {
              tunnel: w847 -> [w856]
              tunnel: [w848] -> w846
              stop <- w849 stop-if-true
              n505 = local read "齿条推拉力(N)"() -> (w854:dbl)
              n506 = Wait Until Next ms Multiple(millisecond multiple=u32 50 ("毫秒倍数")) -> ()  [unwired: 1 out]
              n507 = call <userlib>:"Acm_AxGetCmdVelocity.vi"("AxisHandle"=w856) -> ("Velocity"=w857:dbl, "AxisHandle"=w848:u32)  [unwired: 1 in, 2 out]
              n508 = Equal To 0?(x=w857) -> (x = 0?=w851:bool)
              n509 = Absolute Value(x=w854) -> (abs(x)=w853:dbl)
              n510 = Greater Or Equal?(x=w853, y=1000.0) -> (x >= y?=w850:bool)
              n511 = Or(x=w851, y=w850) -> (x .or. y?=w849:bool)
            }
          }
          frame #4 {
            n512 = while {
              tunnel: w858 -> [w862]
              tunnel: [w861] -> _
              stop <- w860 stop-if-true
              n513 = call "PCI1220U停止.vi"("AxisHandle IN"=w862) -> ("完成"=w860:bool, "AxisHandle OUT"=w861:u32)  [unwired: 9 in]
              n514 = Wait (ms)(milliseconds to wait=u32 50 ("毫秒倍数")) -> ()  [unwired: 1 out]
            }
          }
          frame #5 {
            n515 = local write "旋转齿条轴使能"(TRUE ("旋转齿条轴使能")) -> ()
          }
          frame #6 {
            n516 = Wait Until Next ms Multiple(millisecond multiple=u32 500 ("毫秒倍数")) -> ()  [unwired: 1 out]
          }
          frame #7 {
            n517 = local read "旋转齿条电机"() -> (w866:u32)
            n518 = call <userlib>:"Acm_AxHome.vi"("DirMode"=u32 0, "HomeMode"=u32 11, "AxisHandle"=w866) -> ("AxisHandle"=w865:u32)  [unwired: 1 in, 2 out]
          }
          frame #8 {
            n519 = Wait Until Next ms Multiple(millisecond multiple=u32 100 ("毫秒倍数")) -> ()  [unwired: 1 out]
          }
          frame #9 {
            n520 = while {
              tunnel: w871 -> [w875]
              tunnel: [w874] -> w872
              stop <- w873 stop-if-true
              n521 = call <userlib>:"Acm_AxGetCmdVelocity.vi"("AxisHandle"=w875) -> ("Velocity"=w877:dbl, "AxisHandle"=w874:u32)  [unwired: 1 in, 2 out]
              n522 = Equal To 0?(x=w877) -> (x = 0?=w873:bool)
              n523 = Wait Until Next ms Multiple(millisecond multiple=u32 50 ("毫秒倍数")) -> ()  [unwired: 1 out]
            }
          }
          frame #10 {
            n524 = call "PCI1220U角度置零.vi"("AxisHandle IN"=w879) -> ("AxisHandle OUT"=w878:u32)  [unwired: 10 in]
          }
          frame #11 {
            n525 = while {
              tunnel: [w882] -> w880
              tunnel: w881 -> [w882]
              stop <- w885 stop-if-true
              n526 = Wait Until Next ms Multiple(millisecond multiple=u32 50 ("毫秒倍数")) -> ()  [unwired: 1 out]
              n527 = call "PCI1220U扭矩轴位置模式.vi"("Distance"=15.0, "AxisHandle IN"=w882) -> ("AbsSuccess"=w885:bool)  [unwired: 8 in, 1 out]
            }
          }
          frame #12 {
            n528 = Wait Until Next ms Multiple(millisecond multiple=u32 100 ("毫秒倍数")) -> ()  [unwired: 1 out]
          }
          frame #13 {
            n529 = while {
              tunnel: w888 -> [w892]
              tunnel: [w891] -> w889
              stop <- w890 stop-if-true
              n530 = call <userlib>:"Acm_AxGetCmdVelocity.vi"("AxisHandle"=w892) -> ("Velocity"=w894:dbl, "AxisHandle"=w891:u32)  [unwired: 1 in, 2 out]
              n531 = Equal To 0?(x=w894) -> (x = 0?=w890:bool)
              n532 = Wait Until Next ms Multiple(millisecond multiple=u32 50 ("毫秒倍数")) -> ()  [unwired: 1 out]
            }
          }
          frame #14 {
            n533 = call "PCI1220U角度置零.vi"("AxisHandle IN"=w895) -> ()  [unwired: 10 in, 1 out]
          }
          frame #15 {
            n534 = while {
              tunnel: [w901] -> w896
              stop <- w900 stop-if-true
              n535 = local read "电动缸电机"() -> (w902:u32)
              n536 = Wait Until Next ms Multiple(millisecond multiple=u32 50 ("毫秒倍数")) -> ()  [unwired: 1 out]
              n537 = local read "齿条右极限"() -> (w899:dbl)
              n538 = Add(x=w899, y=-10.0) -> (x+y=w897:dbl)
              n539 = call "PCI1240电动缸位置模式 .vi"("Distance"=w897, "AxisHandle IN"=w902) -> ("AbsSuccess"=w900:bool, "AxisHandle OUT"=w901:u32)  [unwired: 8 in]
            }
          }
          frame #16 {
            n540 = while {
              tunnel: w905 -> [w913]
              tunnel: [w911] -> w904
              stop <- w906 stop-if-true
              n541 = local read "齿条推拉力(N)"() -> (w910:dbl)
              n542 = Wait Until Next ms Multiple(millisecond multiple=u32 50 ("毫秒倍数")) -> ()  [unwired: 1 out]
              n543 = call <userlib>:"Acm_AxGetCmdVelocity.vi"("AxisHandle"=w913) -> ("Velocity"=w914:dbl, "AxisHandle"=w911:u32)  [unwired: 1 in, 2 out]
              n544 = Equal To 0?(x=w914) -> (x = 0?=w907:bool)
              n545 = Greater Or Equal?(x=w910, y=300.0) -> (x >= y?=w908:bool)
              n546 = Or(x=w907, y=w908) -> (x .or. y?=w906:bool)
            }
          }
          frame #17 {
            n547 = while {
              tunnel: w915 -> [w919]
              tunnel: [w918] -> _
              stop <- w917 stop-if-true
              n548 = call "PCI1220U停止.vi"("AxisHandle IN"=w919) -> ("完成"=w917:bool, "AxisHandle OUT"=w918:u32)  [unwired: 9 in]
              n549 = Wait (ms)(milliseconds to wait=u32 50 ("毫秒倍数")) -> ()  [unwired: 1 out]
            }
          }
          frame #18 {
            n550 = local write "工步号"(u32 100 ("工步号")) -> ()
          }
        }
      }
      frame 100 {
        n551 = flat-sequence {
          tunnel: [w954] -> w944
          tunnel: [w952] -> w943
          tunnel: [w946] -> w930
          tunnel: [w945] -> w928
          tunnel: w944 -> [w961]
          tunnel: w943 -> [w958]
          tunnel: ["F:\\报表存储\\" ("字符串")] -> w942
          tunnel: [w961] -> w931
          tunnel: w930 -> [w960]
          tunnel: [w960] -> w929
          tunnel: w928 -> [w959]
          tunnel: [w959] -> w927
          tunnel: [w958] -> w926
          tunnel: w942 -> [w972]
          tunnel: [w980] -> w941
          tunnel: [w977] -> w940
          tunnel: [w976] -> w939
          tunnel: [w975] -> w938
          tunnel: w931 -> [w971]
          tunnel: w929 -> [w970]
          tunnel: w927 -> [w969]
          tunnel: w926 -> [w963]
          tunnel: [w965] -> w925
          tunnel: w941 -> [w987]
          tunnel: [w988] -> w937
          tunnel: w940 -> [w988]
          tunnel: w939 -> [w986]
          tunnel: w938 -> [w985]
          tunnel: [w984] -> w936
          tunnel: [w983] -> w935
          tunnel: w925 -> [w982]
          tunnel: [w982] -> w924
          tunnel: [w995] -> w934
          tunnel: w937 -> [w995]
          tunnel: w936 -> [w994]
          tunnel: [w994] -> w933
          tunnel: [w993] -> w932
          tunnel: w935 -> [w993]
          tunnel: w924 -> [w991]
          tunnel: [w991] -> w923
          tunnel: w934 -> [w998]
          tunnel: w933 -> [w1006]
          tunnel: w932 -> [w1005]
          tunnel: w923 -> [w997]
          tunnel: [w997] -> w922
          tunnel: w922 -> [w1014]
          tunnel: [w1014] -> w921
          tunnel: w921 -> [w1016]
          frame #0 {
            n552 = local read "产品ID"() -> (w953:string)
            n553 = Format Date/Time String(time format string (%c)="%Y%m%d" ("时间格式字符串(%c)")) -> (date/time string=w947:string)  [unwired: 2 in]
            n554 = String Subset(string=w947, offset (0)=4 ("偏移量(0)"), length (rest)=2 ("长度（剩余）")) -> (substring=w946:string)
            n555 = String Subset(string=w947, offset (0)=6 ("偏移量(0)"), length (rest)=2 ("长度（剩余）")) -> (substring=w945:string)
            n556 = call <vilib>:"Trim Whitespace.vi"("string"=w953) -> ("trimmed string"=w952:string)  [unwired: 1 in]
            n557 = String Subset(string=w947, offset (0)=0 ("偏移量(0)"), length (rest)=4 ("长度（剩余）")) -> (substring=w954:string)
          }
          frame #1 {
          }
          frame #2 {
            w964 = "\\" ("字符串")
            n558 = Concatenate Strings(w972, w971, w964, w970, w964, w969, w964, w963, w964) -> (w967:string)
            n559 = Concatenate Strings(w972, w971, w964, w970, w964, w969, w964, w963, w964) -> (w981:string)
            n560 = String To Path(string=w981) -> (path=w980:path)
            n561 = Concatenate Strings(w967, w963, "间隙曲线.JPG" ("字符串")) -> (w978:string)
            n562 = Concatenate Strings(w967, "轴向力曲线数组.txt" ("字符串")) -> (w975:string)
            n563 = Concatenate Strings(w967, "扭动曲线数组.txt" ("字符串")) -> (w976:string)
            n564 = Concatenate Strings(w967, w963, "轴向力曲线.JPG" ("字符串")) -> (w968:string)
            n565 = String To Path(string=w978) -> (path=w977:path)
            n566 = String To Path(string=w968) -> (path=w965:path)
          }
          frame #3 {
            n567 = call <vilib>:"Check if File or Folder Exists.vi"("path"=w987) -> ("file or folder exists?"=w989:bool)  [unwired: 8 in, 2 out]
            n568 = String To Path(string=w985) -> (path=w983:path)
            n569 = String To Path(string=w986) -> (path=w984:path)
            n570 = case shown="假" w989 {
              tunnel: w987 -> [w990 _]
              frame False {
                n571 = Create Folder(path (use dialog)=w990) -> ()  [unwired: 2 in, 3 out]
              }
              frame True {
              }
            }
          }
          frame #4 {
            n572 = local write "选项卡控件"(T1."间隙测量" ("选项卡控件")) -> ()
            n573 = Wait Until Next ms Multiple(millisecond multiple=u32 1000 ("毫秒倍数")) -> ()  [unwired: 1 out]
          }
          frame #5 {
            n574 = disable-structure shown="禁用" {
              disable-tunnel: w998 -> [w1007 _]
              frame Disabled {
                w1011 = T2 2 items=["快速打印", "标准报表", "HTML", "双字节", "Excel"] ("report type (Quick Print)")
                w1010 = T3 1 items=["完整前面板", "前面板可见部分", "图标、说明、前面板和程序框图", "说明信息: 使用前面板", "说明信息: 作为子VI使用", "说明信息: 完整", "说明信息: 自定义"] ("contents (complete front panel)")
                n575 = Current VI's Path() -> (path=w1009:path)
                n576 = call-poly <vilib>:"Easy Print VI Panel or Documentation.vi"("report type (Quick Print)"=w1011, "contents (complete front panel)"=w1010, "VI path"=w1009) -> ("error out"=w1013:errorcluster, "report out"=w1012:refnum<class "NI_report.lvclass">)  [unwired: 1 in, 6 out]
                n577 = call-dynamic "Save Report to File.vi"("report in"=w1012, "report file path"=w1007, "error in (no error)"=w1013) -> ("error out"=→"error out 3":errorcluster)  [unwired: 2 in, 10 out]
              }
              frame Enabled {
              }
            }
            n578 = local read "间隙Y数组"() -> (w1003:dbl[])
            n579 = local read "间隙X数组"() -> (w1004:dbl[])
            n580 = local read "轴向力Y"() -> (w1001:dbl[])
            n581 = local read "轴向力X"() -> (w1002:dbl[])
            n582 = call "导出曲线数组.vi"("file path (dialog if empty)"=w1006, "数组 2"=w1003, "数组"=w1004) -> ()  [unwired: 9 in]
            n583 = call "导出曲线数组.vi"("file path (dialog if empty)"=w1005, "数组 2"=w1001, "数组"=w1002) -> ()  [unwired: 9 in]
            n584 = control-ref of="本VI"() -> (w1000:refnum<vi>)
            n585 = invoke class="VI" method="FP.Get Image"(reference=w1000) -> ("image data"=w999:T4)  [unwired: 5 in, 5 out]
            n586 = call <vilib>:"Write JPEG File.vi"("image data"=w999, "path to JPEG file"=w998) -> ()  [unwired: 8 in, 2 out]
          }
          frame #6 {
            n587 = local write "选项卡控件"(T1."轴向力测量" ("选项卡控件")) -> ()
          }
          frame #7 {
            n588 = control-ref of="本VI"() -> (w1017:refnum<vi>)
            n589 = invoke class="VI" method="FP.Get Image"(reference=w1017) -> ("image data"=w1018:T4)  [unwired: 5 in, 5 out]
            n590 = call <vilib>:"Write JPEG File.vi"("image data"=w1018, "path to JPEG file"=w1016) -> ()  [unwired: 8 in, 2 out]
          }
          frame #8 {
            n591 = local read "联线按钮"() -> (w1019:bool)
            n592 = case shown="真" w1019 {
              frame False {
              }
              frame True {
                n593 = flat-sequence {
                  tunnel: [w1026] -> w1020
                  tunnel: w1020 -> [w1043]
                  frame #0 {
                    n594 = local read "全行程间隙及轴向力合格"() -> (w1021:bool)
                    n595 = local read "单点间隙合格"() -> (w1022:bool)
                    n596 = local read "左全行程间隙"() -> (w1029:dbl)
                    n597 = local read "中间位置间隙"() -> (w1032:dbl)
                    n598 = local read "FGCS"() -> (w1034:string)
                    n599 = local read "员工ID"() -> (w1039:string)
                    n600 = And(x=w1022, y=w1021) -> (x .and. y?=w1023:bool)
                    n601 = local read "KSJJ"() -> (w1036:string)
                    n602 = local read "产品ID"() -> (w1040:string)
                    n603 = Boolean To (0,1)(Boolean=w1023) -> (0, 1=w1038:i16)
                    n604 = Format Date/Time String(time format string (%c)="%Y%m%d%H%M" ("时间格式字符串(%c)")) -> (date/time string=w1035:string)  [unwired: 2 in]
                    n605 = Number To Decimal String(number=w1038, width (-)=i16 1 ("宽度(-)")) -> (decimal integer string=w1024:string)
                    n606 = Number To Fractional String(number=w1029, precision (6)=i16 3 ("精度(6)")) -> (F-format string=w1027:string)  [unwired: 2 in]
                    n607 = Number To Fractional String(number=w1032, precision (6)=i16 3 ("精度(6)")) -> (F-format string=w1028:string)  [unwired: 2 in]
                    n608 = Build Array(w1040, w1039, "1", w1024, w1036, w1035, w1034, "Q14070-Z060A", w1028, w1027) -> (w1026:string[])
                  }
                  frame #1 {
                    n609 = Wait (ms)(milliseconds to wait=u32 500 ("等待时间（毫秒）")) -> ()  [unwired: 1 out]
                    n610 = call "数据库更新.vi"("设备号"="06", "数据"=w1043) -> ()  [unwired: 13 in, 1 out]
                  }
                  frame #2 {
                  }
                }
              }
            }
          }
          frame #9 {
            n611 = local write "产品ID"("") -> ()
            n612 = local write "工步号"(u32 0 ("工步号")) -> ()
          }
        }
      }
    }
    n613 = Wait (ms)(milliseconds to wait=u32 50 ("毫秒倍数")) -> ()  [unwired: 1 out]
    n614 = local read "停止"() -> (w7:bool)
  }
  n615 = while {
    stop <- w1047 stop-if-true
    n616 = event shown="[2] \"参数修改\": 值改变" {
      selector: _ -> [_ _ _ _ _ _ _]
      dyn-events: _ -> [_ _ _ _ _ _ _]
      timeout: 500 -> [_ _ _ _ _ _ _]
      event Timeout {
        n617 = event-data() -> ()  [unwired: 3 out]
      }
      event "停止": Value Change {
        n618 = event-data() -> ()  [unwired: 6 out]
        n619 = flat-sequence {
          frame #0 {
            n620 = Wait (ms)(milliseconds to wait=u32 1000 ("毫秒倍数")) -> ()  [unwired: 1 out]
          }
          frame #1 {
            n621 = Quit LabVIEW(quit? (T)=TRUE ("停止？(T)")) -> ()
          }
        }
      }
      event "参数修改": Value Change {
        n622 = event-data() -> ()  [unwired: 6 out]
        n623 = while {
          i -> [w1099]
          stop <- w1098 stop-if-true
          n624 = local read "型号数量"() -> (w1100:i32)
          n625 = local read "参数浏览表"() -> (w1101:string[][])
          n626 = Greater Or Equal?(x=w1099, y=w1100) -> (x >= y?=w1098:bool)
          n627 = Wait Until Next ms Multiple(millisecond multiple=u32 50 ("毫秒倍数")) -> ()  [unwired: 1 out]
          n628 = Index Array(array=w1101, index (col)=w1099) -> (element=w1086:string[])  [unwired: 1 in]
          n629 = Index Array(array=w1086, index #1=0 ("索引"), index #2=2 ("索引"), index #3=3 ("索引"), index #4=4 ("索引"), index #5=5 ("索引"), index #6=6 ("索引"), index #7=7 ("索引"), index #8=8 ("索引"), index #9=9 ("索引"), index #10=10 ("索引"), index #11=11 ("索引"), index #12=12 ("索引"), index #13=13 ("索引"), index #14=14 ("索引"), index #15=15 ("索引"), index #16=16 ("索引"), index #17=17 ("索引"), index #18=18 ("索引"), index #19=19 ("索引"), index #20=20 ("索引")) -> (element #1=w1053:string, element #2=w1082:string, element #3=w1081:string, element #4=w1080:string, element #5=w1079:string, element #6=w1078:string, element #7=w1077:string, element #8=w1076:string, element #9=w1075:string, element #10=w1074:string, element #11=w1073:string, element #12=w1068:string, element #13=w1067:string, element #14=w1066:string, element #15=w1065:string, element #16=w1064:string, element #17=w1059:string, element #18=w1058:string, element #19=w1057:string, element #20=w1052:string)
          n630 = call "创建文本"("测头机构轴移动速度"=w1082, "测头机构轴检测位"=w1081, "测头机构轴待检位"=w1080, "测头机构轴后退位"=w1079, "齿条移动速度"=w1078, "齿条左极限"=w1077, "齿条右极限"=w1076, "旋转齿条轴找帽转速"=w1075, "旋转齿条轴测量转速"=w1074, "测量点扭矩"=w1073, "总行程最大值"=w1067, "总行程最小值"=w1068, "最大轴向力"=w1066, "轴向力波动"=w1065, "平均轴向力最小值"=w1064, "平均轴向力最大值"=w1059, "总圈数最小值"=w1058, "总圈数最大值"=w1057, "中间位置"=w1052, "产品型号"=w1053) -> ("Result"=w1072:string)  [unwired: 6 in, 1 out]
          n631 = local read "ADODB._Connection Out 2"() -> (w1071:refnum<k7>)
          n632 = call "SQL Execute.vi"("Command Text"=w1072, "ADODB._Connection In"=w1071) -> ("error out"=w1084:errorcluster, "ADODB._Connection Out"=w1085:refnum<k7>)  [unwired: 6 in, 2 out]
          n633 = call "ADO Connection Close.vi"("error in (no error)"=w1084, "ADODB._Connection In"=w1085) -> ("error out"=→"error out":errorcluster)  [unwired: 8 in, 1 out]
        }
      }
      event "参数查询": Value Change {
        n634 = event-data() -> ()  [unwired: 6 out]
        n635 = flat-sequence {
          tunnel: [w1114] -> w1107
          tunnel: [w1113] -> w1106
          tunnel: [w1112] -> w1103
          tunnel: w1107 -> [w1118]
          tunnel: w1106 -> [w1120]
          tunnel: [w1120] -> w1105
          tunnel: [w1119] -> w1104
          tunnel: w1103 -> [w1119]
          tunnel: w1105 -> [_]
          tunnel: w1104 -> [_]
          frame #0 {
            n636 = call-poly <vilib>:"Read From Spreadsheet File.vi"("file path (dialog if empty)"=path "D:/Q14070-Z060人机界面/参数/参数项.txt") -> ("first row"=w1108:string[])  [unwired: 6 in, 4 out]
            n637 = property on="参数浏览表" class="Tbl (严格)"("Row Headers[]"=w1108) -> ()  [unwired: 2 in, 2 out]
          }
          frame #1 {
            n638 = local read "ADODB._Connection Out 2"() -> (w1111:refnum<k7>)
            n639 = call "SQL Execute.vi"("Command Text"="SELECT * FROM 测试参数表;", "ADODB._Connection In"=w1111) -> ("error out"=w1112:errorcluster, "Data"=w1116:string[][], "ADODB._Connection Out"=w1113:refnum<k7>)  [unwired: 6 in, 1 out]
            n640 = Transpose 2D Array(2D array=w1116) -> (transposed array=w1114:string[][])
            n641 = Index Array(array=w1114, index (row)=0 ("索引 (行)")) -> (element=w1115:string[])  [unwired: 1 in]
            n642 = property on="参数浏览表" class="Tbl (严格)"("Column Headers[]"=w1115) -> ()  [unwired: 2 in, 2 out]
          }
          frame #2 {
            n643 = local write "参数浏览表"(w1118) -> ()
          }
          frame #3 {
          }
        }
      }
      event "传感器参数保存": Value Change {
        n644 = event-data() -> ()  [unwired: 6 out]
        n645 = flat-sequence {
          tunnel: [w1146] -> w1143
          tunnel: [w1145] -> w1142
          tunnel: [w1144] -> w1141
          tunnel: [w1152] -> w1140
          tunnel: w1143 -> [w1152]
          tunnel: [w1151] -> w1139
          tunnel: w1142 -> [w1151]
          tunnel: [w1150] -> w1138
          tunnel: w1141 -> [w1150]
          tunnel: [w1149] -> w1137
          tunnel: [w1148] -> w1136
          tunnel: [w1147] -> w1135
          tunnel: [w1153] -> w1134
          tunnel: [w1159] -> w1133
          tunnel: w1140 -> [w1159]
          tunnel: [w1158] -> w1132
          tunnel: w1139 -> [w1158]
          tunnel: w1138 -> [w1157]
          tunnel: [w1157] -> w1131
          tunnel: [w1156] -> w1130
          tunnel: w1137 -> [w1156]
          tunnel: [w1155] -> w1129
          tunnel: w1136 -> [w1155]
          tunnel: [w1154] -> w1128
          tunnel: w1135 -> [w1154]
          tunnel: w1134 -> [w1178]
          tunnel: [w1178] -> w1127
          tunnel: w1133 -> [w1177]
          tunnel: w1132 -> [w1170]
          tunnel: w1131 -> [w1169]
          tunnel: w1130 -> [w1163]
          tunnel: w1129 -> [w1162]
          tunnel: w1128 -> [w1168]
          tunnel: [w1167] -> w1126
          tunnel: [w1166] -> w1125
          tunnel: [w1165] -> w1124
          tunnel: [w1161] -> w1123
          tunnel: [w1160] -> w1122
          tunnel: [w1164] -> w1121
          tunnel: w1127 -> [w1186]
          tunnel: w1126 -> [w1185]
          tunnel: w1125 -> [w1184]
          tunnel: w1124 -> [w1183]
          tunnel: w1123 -> [w1182]
          tunnel: w1122 -> [w1181]
          tunnel: w1121 -> [w1180]
          frame #0 {
            n646 = local read "齿条推拉力零点偏移"() -> (w1145:dbl)
            n647 = local read "间隙位移零点偏移"() -> (w1146:dbl)
            n648 = local read "齿条扭矩零点偏移"() -> (w1144:dbl)
          }
          frame #1 {
            n649 = local read "齿条推拉力比例偏移"() -> (w1148:dbl)
            n650 = local read "间隙位移比例偏移"() -> (w1149:dbl)
            n651 = local read "齿条扭矩比例偏移"() -> (w1147:dbl)
          }
          frame #2 {
            n652 = local read "ADODB._Connection Out 2"() -> (w1153:refnum<k7>)
          }
          frame #3 {
            n653 = Number To Fractional String(number=w1177, precision (6)=i16 2 ("精度(6)")) -> (F-format string=w1167:string)  [unwired: 2 in]
            n654 = Number To Fractional String(number=w1169, precision (6)=i16 2 ("精度(6)")) -> (F-format string=w1165:string)  [unwired: 2 in]
            n655 = Number To Fractional String(number=w1168, precision (6)=i16 2 ("精度(6)")) -> (F-format string=w1164:string)  [unwired: 2 in]
            n656 = Number To Fractional String(number=w1170, precision (6)=i16 2 ("精度(6)")) -> (F-format string=w1166:string)  [unwired: 2 in]
            n657 = Number To Fractional String(number=w1163, precision (6)=i16 2 ("精度(6)")) -> (F-format string=w1161:string)  [unwired: 2 in]
            n658 = Number To Fractional String(number=w1162, precision (6)=i16 2 ("精度(6)")) -> (F-format string=w1160:string)  [unwired: 2 in]
          }
          frame #4 {
            n659 = call "创建文本3"("4"=w1182, "6"=w1180, "1"=w1185, "2"=w1184, "3"=w1183, "5"=w1181) -> ("Result"=w1187:string)  [unwired: 8 in, 1 out]
            n660 = call "SQL Execute.vi"("Command Text"=w1187, "ADODB._Connection In"=w1186) -> ("error out"=→"error out 4":errorcluster)  [unwired: 6 in, 3 out]
          }
        }
      }
      event "产品ID": Value Change {
        n661 = event-data() -> ()  [unwired: 7 out]
        n662 = Format Date/Time String(time format string (%c)="%Y%m%d%H%M" ("时间格式字符串(%c)")) -> (date/time string=w1188:string)  [unwired: 2 in]
        n663 = local write "KSJJ"(w1188) -> ()
      }
      event "电动缸回零": Mouse Down {
        n664 = event-data() -> ()  [unwired: 6 out]
        n665 = stacked-sequence {
          frame #0 {
            n666 = flat-sequence {
              tunnel: [w1208] -> w1197
              tunnel: [w1201] -> w1194
              tunnel: w1197 -> [w1211]
              tunnel: [w1211] -> w1196
              tunnel: [w1209] -> w1195
              tunnel: w1194 -> [w1209]
              tunnel: w1196 -> [w1213]
              tunnel: [w1213] -> w1198
              tunnel: w1195 -> [w1212]
              tunnel: [w1212] -> w1193
              tunnel: w1198 -> [w1224]
              tunnel: w1193 -> [w1223]
              tunnel: [w1222] -> w1192
              tunnel: w1192 -> [w1226]
              tunnel: [w1225] -> w1191
              tunnel: w1191 -> [w1234]
              frame #0 {
                n667 = local write "电动缸速度(mm/s)"(15.0 ("电动缸速度(mm/s)")) -> ()
                n668 = local write "测头机构轴速度(mm/s)"(10.0 ("电动缸速度(mm/s)")) -> ()
              }
              frame #1 {
                n669 = local read "测头机构电机"() -> (w1205:u32)
                n670 = local read "电动缸电机"() -> (w1202:u32)
                n671 = call <userlib>:"Acm_AxHome.vi"("DirMode"=u32 0, "HomeMode"=u32 11, "AxisHandle"=w1205) -> ("AxisHandle"=w1208:u32)  [unwired: 1 in, 2 out]
                n672 = call <userlib>:"Acm_AxHome.vi"("DirMode"=u32 1, "HomeMode"=u32 11, "AxisHandle"=w1202) -> ("AxisHandle"=w1201:u32)  [unwired: 1 in, 2 out]
              }
              frame #2 {
                n673 = Wait Until Next ms Multiple(millisecond multiple=u32 100 ("毫秒倍数")) -> ()  [unwired: 1 out]
              }
              frame #3 {
                n674 = while {
                  tunnel: w1213 -> [w1221]
                  stop <- w1219 stop-if-true
                  n675 = call <userlib>:"Acm_AxGetCmdVelocity.vi"("AxisHandle"=w1221) -> ("Velocity"=w1220:dbl)  [unwired: 1 in, 3 out]
                  n676 = Wait Until Next ms Multiple(millisecond multiple=u32 50 ("毫秒倍数")) -> ()  [unwired: 1 out]
                  n677 = Equal To 0?(x=w1220) -> (x = 0?=w1219:bool)
                }
                n678 = while {
                  tunnel: w1212 -> [w1217]
                  stop <- w1215 stop-if-true
                  n679 = call <userlib>:"Acm_AxGetCmdVelocity.vi"("AxisHandle"=w1217) -> ("Velocity"=w1216:dbl)  [unwired: 1 in, 3 out]
                  n680 = Wait Until Next ms Multiple(millisecond multiple=u32 50 ("毫秒倍数")) -> ()  [unwired: 1 out]
                  n681 = Equal To 0?(x=w1216) -> (x = 0?=w1215:bool)
                }
              }
              frame #4 {
                n682 = call "PCI1220U角度置零.vi"("AxisHandle IN"=w1224) -> ()  [unwired: 10 in, 1 out]
                n683 = call "PCI1220U角度置零.vi"("AxisHandle IN"=w1223) -> ("AxisHandle OUT"=w1222:u32)  [unwired: 10 in]
              }
              frame #5 {
                n684 = while {
                  tunnel: [w1232] -> w1225
                  tunnel: w1226 -> [w1227]
                  stop <- w1231 stop-if-true
                  n685 = Wait Until Next ms Multiple(millisecond multiple=u32 50 ("毫秒倍数")) -> ()  [unwired: 1 out]
                  n686 = local read "齿条右极限"() -> (w1230:dbl)
                  n687 = Add(x=w1230, y=-10.0) -> (x+y=w1228:dbl)
                  n688 = call "PCI1240电动缸位置模式 .vi"("Distance"=w1228, "AxisHandle IN"=w1227) -> ("AbsSuccess"=w1231:bool, "AxisHandle OUT"=w1232:u32)  [unwired: 8 in]
                }
              }
              frame #6 {
                n689 = while {
                  tunnel: w1234 -> [w1238]
                  stop <- w1236 stop-if-true
                  n690 = call <userlib>:"Acm_AxGetCmdVelocity.vi"("AxisHandle"=w1238) -> ("Velocity"=w1237:dbl)  [unwired: 1 in, 3 out]
                  n691 = Wait Until Next ms Multiple(millisecond multiple=u32 50 ("毫秒倍数")) -> ()  [unwired: 1 out]
                  n692 = Equal To 0?(x=w1237) -> (x = 0?=w1236:bool)
                }
              }
            }
          }
          frame #1 {
            n693 = flat-sequence {
              tunnel: [w1250] -> w1245
              tunnel: w1245 -> [w1252]
              tunnel: [w1252] -> w1244
              tunnel: w1244 -> [w1253]
              tunnel: [w1253] -> w1243
              tunnel: w1243 -> [w1259]
              tunnel: [w1258] -> w1240
              tunnel: w1240 -> [w1261]
              tunnel: [w1261] -> w1239
              tunnel: w1239 -> [w1263]
              tunnel: [w1262] -> w1242
              tunnel: w1242 -> [w1269]
              tunnel: [w1269] -> w1241
              tunnel: w1241 -> [w1274]
              frame #0 {
                n694 = local write "旋转伺服速度(°/s)"(5.0 ("电动缸速度(mm/s)")) -> ()
              }
              frame #1 {
                n695 = local read "旋转齿条电机"() -> (w1247:u32)
                n696 = call <userlib>:"Acm_AxHome.vi"("DirMode"=u32 0, "HomeMode"=u32 11, "AxisHandle"=w1247) -> ("AxisHandle"=w1250:u32)  [unwired: 1 in, 2 out]
              }
              frame #2 {
                n697 = Wait Until Next ms Multiple(millisecond multiple=u32 100 ("毫秒倍数")) -> ()  [unwired: 1 out]
              }
              frame #3 {
                n698 = while {
                  tunnel: w1253 -> [w1257]
                  stop <- w1255 stop-if-true
                  n699 = call <userlib>:"Acm_AxGetCmdVelocity.vi"("AxisHandle"=w1257) -> ("Velocity"=w1256:dbl)  [unwired: 1 in, 3 out]
                  n700 = Wait Until Next ms Multiple(millisecond multiple=u32 50 ("毫秒倍数")) -> ()  [unwired: 1 out]
                  n701 = Equal To 0?(x=w1256) -> (x = 0?=w1255:bool)
                }
              }
              frame #4 {
                n702 = call "PCI1220U角度置零.vi"("AxisHandle IN"=w1259) -> ("AxisHandle OUT"=w1258:u32)  [unwired: 10 in]
              }
              frame #5 {
                n703 = Wait (ms)(milliseconds to wait=u32 100 ("等待时间（毫秒）")) -> ()  [unwired: 1 out]
              }
              frame #6 {
                n704 = while {
                  tunnel: [w1267] -> w1262
                  tunnel: w1263 -> [w1264]
                  stop <- w1266 stop-if-true
                  n705 = Wait Until Next ms Multiple(millisecond multiple=u32 50 ("毫秒倍数")) -> ()  [unwired: 1 out]
                  n706 = call "PCI1220U扭矩轴位置模式.vi"("Distance"=15.0, "AxisHandle IN"=w1264) -> ("AbsSuccess"=w1266:bool, "AxisHandle OUT"=w1267:u32)  [unwired: 8 in]
                }
              }
              frame #7 {
                n707 = while {
                  tunnel: w1269 -> [w1272]
                  stop <- w1270 stop-if-true
                  n708 = call <userlib>:"Acm_AxGetCmdVelocity.vi"("AxisHandle"=w1272) -> ("Velocity"=w1273:dbl)  [unwired: 1 in, 3 out]
                  n709 = Wait Until Next ms Multiple(millisecond multiple=u32 50 ("毫秒倍数")) -> ()  [unwired: 1 out]
                  n710 = Equal To 0?(x=w1273) -> (x = 0?=w1270:bool)
                }
              }
              frame #8 {
                n711 = call "PCI1220U角度置零.vi"("AxisHandle IN"=w1274) -> ()  [unwired: 10 in, 1 out]
              }
            }
          }
          frame #2 {
            n712 = flat-sequence {
              frame #0 {
                n713 = while {
                  stop <- w1278 stop-if-true
                  n714 = local read "电动缸回零"() -> (w1279:bool)
                  n715 = local write "回零完成"(TRUE ("回零完成")) -> ()
                  n716 = local write "电动缸回零"(FALSE ("电动缸回零")) -> ()
                  n717 = Wait Until Next ms Multiple(millisecond multiple=u32 50 ("毫秒倍数")) -> ()  [unwired: 1 out]
                  n718 = Not(x=w1279) -> (.not. x?=w1278:bool)
                }
              }
            }
          }
        }
        n719 = Wait Until Next ms Multiple(millisecond multiple=u32 50 ("毫秒倍数")) -> ()  [unwired: 1 out]
      }
    }
    n720 = Wait (ms)(milliseconds to wait=u32 50 ("毫秒倍数")) -> ()  [unwired: 1 out]
    n721 = local read "停止"() -> (w1047:bool)
  }
  n722 = call "PCI1240电动缸位置模式 .vi"() -> ()  [unwired: 10 in, 2 out]
  n723 = while {
    stop <- w1281 stop-if-true
    n724 = stacked-sequence {
      frame #0 {
        n725 = flat-sequence {
          frame #0 {
          }
          frame #1 {
            n726 = First Call?() -> (First Call?: T/F=w1282:bool)
            n727 = case shown="真" w1282 {
              frame False {
              }
              frame True {
                n728 = call "员工管理测试程序.vi"() -> ("员工姓名"=w1284:string, "员工ID"=w1283:string)  [unwired: 10 in]
                n729 = local write "员工ID"(w1283) -> ()
                n730 = local write "员工姓名"(w1284) -> ()
              }
            }
          }
          frame #2 {
          }
          frame #3 {
          }
          frame #4 {
          }
          frame #5 {
          }
          frame #6 {
          }
        }
      }
      frame #1 {
        n731 = flat-sequence {
          frame #0 {
            n732 = property on="型号选择" class="Ring (严格)"() -> ("RingText.Text"=w1285:string)  [unwired: 2 in, 2 out]
            n733 = case shown="\"J728\"" w1285 {
              frame "J706" {
                w1286 = FALSE ("可见")
                w1287 = TRUE ("可见")
                n734 = property on="左180°内全行程间隙" class="DigNum (严格)"("Visible"=w1287) -> ()  [unwired: 2 in, 2 out]
                n735 = property on="左180°外全行程间隙" class="DigNum (严格)"("Visible"=w1287) -> ()  [unwired: 2 in, 2 out]
                n736 = property on="右180°外全行程间隙" class="DigNum (严格)"("Visible"=w1287) -> ()  [unwired: 2 in, 2 out]
                n737 = property on="右180°内全行程间隙" class="DigNum (严格)"("Visible"=w1287) -> ()  [unwired: 2 in, 2 out]
                n738 = property on="左全行程间隙" class="DigNum (严格)"("Visible"=w1286) -> ()  [unwired: 2 in, 2 out]
                n739 = property on="右全行程间隙" class="DigNum (严格)"("Visible"=w1286) -> ()  [unwired: 2 in, 2 out]
              }
              frame "J728" {
                w1288 = FALSE ("可见")
                w1289 = TRUE ("可见")
                n740 = property on="左180°内全行程间隙" class="DigNum (严格)"("Visible"=w1289) -> ()  [unwired: 2 in, 2 out]
                n741 = property on="左180°外全行程间隙" class="DigNum (严格)"("Visible"=w1289) -> ()  [unwired: 2 in, 2 out]
                n742 = property on="右180°外全行程间隙" class="DigNum (严格)"("Visible"=w1289) -> ()  [unwired: 2 in, 2 out]
                n743 = property on="右180°内全行程间隙" class="DigNum (严格)"("Visible"=w1289) -> ()  [unwired: 2 in, 2 out]
                n744 = property on="左全行程间隙" class="DigNum (严格)"("Visible"=w1288) -> ()  [unwired: 2 in, 2 out]
                n745 = property on="右全行程间隙" class="DigNum (严格)"("Visible"=w1288) -> ()  [unwired: 2 in, 2 out]
              }
              frame "J709", Default {
                w1290 = TRUE ("可见")
                w1291 = FALSE ("可见")
                n746 = property on="左180°内全行程间隙" class="DigNum (严格)"("Visible"=w1291) -> ()  [unwired: 2 in, 2 out]
                n747 = property on="左180°外全行程间隙" class="DigNum (严格)"("Visible"=w1291) -> ()  [unwired: 2 in, 2 out]
                n748 = property on="右180°外全行程间隙" class="DigNum (严格)"("Visible"=w1291) -> ()  [unwired: 2 in, 2 out]
                n749 = property on="右180°内全行程间隙" class="DigNum (严格)"("Visible"=w1291) -> ()  [unwired: 2 in, 2 out]
                n750 = property on="左全行程间隙" class="DigNum (严格)"("Visible"=w1290) -> ()  [unwired: 2 in, 2 out]
                n751 = property on="右全行程间隙" class="DigNum (严格)"("Visible"=w1290) -> ()  [unwired: 2 in, 2 out]
              }
            }
          }
          frame #1 {
            (unwired) string[] ["I急停按钮", "I自动旋钮", "I启动按钮", "I备用按钮", "I复位按钮", "I上阻挡器放行", "I下阻挡器放行", "I进支线按钮"] ("I0说明")
            (unwired) string[] ["I出支线按钮", "I主线顶升按钮", "I主线下降按钮", "I支线顶升按钮", "I支线下降按钮", "I气压报警", "未使用", "未使用"] ("I0说明")
            n752 = local read "间隙位移(mm)"() -> (w1294:dbl)
            n753 = Greater Or Equal?(x=w1294, y=7.0) -> (x >= y?=w1292:bool)
            n754 = case shown="真" w1292 {
              frame False {
              }
              frame True {
                n755 = local write "测头机构轴使能"(FALSE ("测头机构轴使能")) -> ()
              }
            }
          }
          frame #2 {
            (unwired) string[] ["I电动缸SRDY", "I电动缸ZSPD", "I电动缸ALRM", "I间隙进给SRDY", "I间隙进给ZSPD", "I间隙进给ALRM", "I间隙旋转SRPD", "I间隙旋转ZSPD"] ("I0说明")
            n756 = local read "测头机构轴位置(mm)"() -> (w1298:dbl)
            n757 = Greater Or Equal?(x=w1298, y=90.0) -> (x >= y?=w1296:bool)
            n758 = case shown="假" w1296 {
              frame False {
                w1299 = T5."Enabled" ("禁用")
                n759 = property on="测头气缸左移" class="Bool (严格)"("DisabledEnum"=w1299) -> ()  [unwired: 2 in, 2 out]
                n760 = property on="测头气缸右移" class="Bool (严格)"("DisabledEnum"=w1299) -> ()  [unwired: 2 in, 2 out]
                n761 = property on="测头气缸左移" class="Bool"("DisabledEnum"=w1299) -> ()  [unwired: 2 in, 2 out]
                n762 = property on="测头气缸右移" class="Bool"("DisabledEnum"=w1299) -> ()  [unwired: 2 in, 2 out]
              }
              frame True {
                w1300 = T5."Disabled" ("禁用")
                w1301 = FALSE ("测头气缸右移")
                n763 = local write "测头气缸右移"(w1301) -> ()
                n764 = local write "测头气缸左移"(w1301) -> ()
                n765 = property on="测头气缸左移" class="Bool (严格)"("DisabledEnum"=w1300) -> ()  [unwired: 2 in, 2 out]
                n766 = property on="测头气缸右移" class="Bool (严格)"("DisabledEnum"=w1300) -> ()  [unwired: 2 in, 2 out]
                n767 = property on="测头气缸左移" class="Bool"("DisabledEnum"=w1300) -> ()  [unwired: 2 in, 2 out]
                n768 = property on="测头气缸右移" class="Bool"("DisabledEnum"=w1300) -> ()  [unwired: 2 in, 2 out]
              }
            }
          }
          frame #3 {
            (unwired) string[] ["I间隙旋转ALRM", "I扭矩旋转SRPD", "I扭矩旋转ZSPD", "I扭矩旋转ALRM", "I拧紧机合格", "I拧紧机不合格", "I拧紧机报警", "未使用"] ("I0说明")
          }
        }
      }
      frame #2 {
        n769 = flat-sequence {
          frame #0 {
            (unwired) string[] ["I自制气缸进位", "I自制气缸原位", "I上工位检测", "I本工位检测", "I下工位检测", "I主线顶升上位", "I主线顶升下位", "I支线顶升上位"] ("I0说明")
          }
          frame #1 {
            (unwired) string[] ["I支线顶升下位", "I支线进到位", "I支线退到位", "I位移气缸原位", "I位移气缸进位", "I拧紧机在位", "I电动缸原位", "I电动缸进位"] ("I0说明")
          }
          frame #2 {
            (unwired) string[] ["未使用", "未使用", "未使用", "未使用", "未使用", "未使用", "未使用", "未使用"] ("I0说明")
          }
          frame #3 {
            (unwired) string[] ["未使用", "未使用", "未使用", "未使用", "未使用", "未使用", "未使用", "未使用"] ("I0说明")
          }
        }
        n770 = local read "下工位测试H"() -> (w1303:bool)
        n771 = local read "下工位备料H"() -> (w1302:bool)
        n772 = local read "下工位自动H"() -> (w1304:bool)
        n773 = local write "下工位备料"(w1302) -> ()
        n774 = local write "下工位测试"(w1303) -> ()
        n775 = local write "下工位自动"(w1304) -> ()
      }
      frame #3 {
        n776 = local read "工步号"() -> (w1308:u32)
        n777 = local read "报警"() -> (w1306:dbl)
        n778 = case shown="50" w1308 {
          tunnel: [w1319 "请取胶瓶" ("工步描述") "请取扳手加力" ("工步描述") "灵敏度测试中" ("工步描述") "有油刚度测试中" ("工步描述") "点击启动按钮进行测试" ("工步描述") "电动缸前进找中" ("工步描述") "气缸右移" ("工步描述") "电动缸前进找中" ("工步描述") "找中结束开始测间隙" ("工步描述") "力特性试验中" ("工步描述") "轴向力测试中" ("工步描述") "探头气缸左移，电动缸后退" ("工步描述") "等待放行" ("工步描述") "电动缸回零" ("工步描述") "力特性试验完成" ("工步描述") "套好输出轴把手，按启动按钮，做回正力试验" ("工步描述") "回正力试验中" ("工步描述") "试验完成，将把手拉回，取下油管，按顶升按钮" ("工步描述") "拆下锁紧螺母和输入轴万向节，按顶升按钮" ("工步描述")] -> w1307
          frame 0, Default {
            n779 = local read "联线按钮"() -> (w1318:bool)
            n780 = case shown="假" w1318 {
              tunnel: ["等待工件" ("工步描述") "等待扫描条码" ("工步描述")] -> w1319
              frame False {
              }
              frame True {
              }
            }
          }
          frame 1 {
          }
          frame 2 {
          }
          frame 3 {
          }
          frame 4 {
          }
          frame 6 {
          }
          frame 7 {
          }
          frame 10 {
          }
          frame 15 {
          }
          frame 20 {
          }
          frame 30 {
          }
          frame 40 {
          }
          frame 45 {
          }
          frame 100 {
          }
          frame 50 {
          }
          frame 55 {
          }
          frame 60 {
          }
          frame 70 {
          }
          frame 80 {
          }
          frame 56 {
          }
        }
        "工步提示" <- w1307
        n781 = case shown="9" w1306 {
          tunnel: [_ "探头气缸不在原位" "操作步骤错误请取胶瓶" "操作步骤错误请加力" "急停被按下" "气压报警" "电动缸伺服报警" "旋转伺服报警" "测头伺服报警" "操作步骤错误请点标后放行"] -> w1305
          frame 0, Default {
          }
          frame 1 {
          }
          frame 2 {
          }
          frame 3 {
          }
          frame 4 {
          }
          frame 5 {
          }
          frame 6 {
          }
          frame 7 {
          }
          frame 8 {
          }
          frame 9 {
          }
        }
        n782 = local write "报警提示"(w1305) -> ()
      }
      frame #4 {
        n783 = local read "急停"() -> (w1341:bool)
        n784 = local read "红灯"() -> (w1343:bool)
        n785 = local read "复位"() -> (w1344:bool)
        n786 = local read "复位"() -> (w1346:bool)
        n787 = local read "红灯"() -> (w1345:bool)
        n788 = case shown="真" w1341 {
          frame False {
            "红灯" <- TRUE ("红灯")
          }
          frame True {
            n789 = local write "红灯"(FALSE ("红灯")) -> ()
          }
        }
        n790 = Or(x=w1343, y=w1344) -> (x .or. y?=w1342:bool)
        n791 = case shown="真" w1342 {
          frame False {
          }
          frame True {
            n792 = local write "回零完成"(FALSE ("夹头夹紧控制")) -> ()
          }
        }
        n793 = local read "停止"() -> (w1348:bool)
        n794 = Compound Arithmetic op=OR(w1346, w1348, w1345) -> (w1347:bool)
        n795 = case shown="真" w1347 {
          frame False {
          }
          frame True {
            n796 = local read "测头机构电机"() -> (w1352:u32)
            n797 = local read "旋转齿条电机"() -> (w1353:u32)
            n798 = local read "电动缸电机"() -> (w1354:u32)
            n799 = call "PCI1220U停止.vi"("AxisHandle IN"=w1353) -> ()  [unwired: 9 in, 2 out]
            n800 = call "PCI1220U停止.vi"("AxisHandle IN"=w1354) -> ()  [unwired: 9 in, 2 out]
            n801 = call "PCI1220U停止.vi"("AxisHandle IN"=w1352) -> ()  [unwired: 9 in, 2 out]
          }
        }
      }
      frame #5 {
        n802 = local read "齿条扭矩(Nm)"() -> (w1357:dbl)
        n803 = local read "黄灯"() -> (w1355:bool)
        n804 = local read "旋转齿条轴左转"() -> (w1363:bool)
        n805 = Absolute Value(x=w1357) -> (abs(x)=w1362:dbl)
        n806 = local read "旋转齿条轴右转"() -> (w1358:bool)
        n807 = Not(x=w1363) -> (.not. x?=w1359:bool)
        n808 = Less?(x=w1362, y=20.0) -> (x < y?=w1360:bool)
        n809 = Compound Arithmetic op=AND(w1358, w1359, w1360, w1355) -> (w1356:bool)
        n810 = case shown="真" w1356 {
          frame False {
          }
          frame True {
            n811 = flat-sequence {
              tunnel: [w1367] -> w1365
              tunnel: w1365 -> [w1369]
              tunnel: [w1369] -> w1364
              tunnel: w1364 -> [w1380]
              frame #0 {
                n812 = local read "旋转齿条电机"() -> (w1366:u32)
                n813 = call "PCI1220U运行.vi"("方向"=enum32{"Negative", "Positive"}."Negative" ("Direction"), "AxisHandle IN"=w1366) -> ("AxisHandle OUT"=w1367:u32)  [unwired: 9 in]
              }
              frame #1 {
                n814 = while {
                  stop <- w1373 stop-if-true
                  n815 = Wait (ms)(milliseconds to wait=u32 50 ("毫秒倍数")) -> ()  [unwired: 1 out]
                  n816 = local read "齿条扭矩(Nm)"() -> (w1378:dbl)
                  n817 = local read "旋转齿条轴右转"() -> (w1375:bool)
                  n818 = local read "红灯"() -> (w1370:bool)
                  n819 = local read "复位"() -> (w1371:bool)
                  n820 = Absolute Value(x=w1378) -> (abs(x)=w1377:dbl)
                  n821 = Not(x=w1375) -> (.not. x?=w1372:bool)
                  n822 = Greater?(x=w1377, y=10.0) -> (0:w1374:bool)
                  n823 = Compound Arithmetic op=OR(w1374, w1372, w1371, w1370) -> (w1373:bool)
                }
              }
              frame #2 {
                n824 = call "PCI1220U停止.vi"("AxisHandle IN"=w1380) -> ()  [unwired: 9 in, 2 out]
              }
            }
          }
        }
      }
      frame #6 {
        n825 = local read "齿条扭矩(Nm)"() -> (w1385:dbl)
        n826 = local read "旋转齿条轴右转"() -> (w1389:bool)
        n827 = Absolute Value(x=w1385) -> (abs(x)=w1384:dbl)
        n828 = local read "旋转齿条轴左转"() -> (w1387:bool)
        n829 = local read "黄灯"() -> (w1381:bool)
        n830 = Not(x=w1389) -> (.not. x?=w1386:bool)
        n831 = Less?(x=w1384, y=20.0) -> (x < y?=w1382:bool)
        n832 = Compound Arithmetic op=AND(w1387, w1386, w1382, w1381) -> (w1388:bool)
        n833 = case shown="真" w1388 {
          frame False {
          }
          frame True {
            n834 = flat-sequence {
              tunnel: [w1393] -> w1391
              tunnel: w1391 -> [w1395]
              tunnel: [w1395] -> w1390
              tunnel: w1390 -> [w1406]
              frame #0 {
                n835 = local read "旋转齿条电机"() -> (w1392:u32)
                n836 = call "PCI1220U运行.vi"("方向"=enum32{"Negative", "Positive"}."Positive" ("Direction"), "AxisHandle IN"=w1392) -> ("AxisHandle OUT"=w1393:u32)  [unwired: 9 in]
              }
              frame #1 {
                n837 = while {
                  stop <- w1398 stop-if-true
                  n838 = Wait (ms)(milliseconds to wait=u32 50 ("毫秒倍数")) -> ()  [unwired: 1 out]
                  n839 = local read "齿条扭矩(Nm)"() -> (w1404:dbl)
                  n840 = local read "旋转齿条轴左转"() -> (w1401:bool)
                  n841 = local read "红灯"() -> (w1396:bool)
                  n842 = local read "复位"() -> (w1397:bool)
                  n843 = Absolute Value(x=w1404) -> (abs(x)=w1403:dbl)
                  n844 = Not(x=w1401) -> (.not. x?=w1399:bool)
                  n845 = Greater?(x=w1403, y=10.0) -> (0:w1400:bool)
                  n846 = Compound Arithmetic op=OR(w1397, w1396, w1400, w1399) -> (w1398:bool)
                }
              }
              frame #2 {
                n847 = call "PCI1220U停止.vi"("AxisHandle IN"=w1406) -> ()  [unwired: 9 in, 2 out]
              }
            }
          }
        }
      }
      frame #7 {
        n848 = local read "齿条推拉力(N)"() -> (w1411:dbl)
        n849 = local read "电动缸前进"() -> (w1408:bool)
        n850 = local read "电动缸后退"() -> (w1407:bool)
        n851 = Absolute Value(x=w1411) -> (abs(x)=w1415:dbl)
        n852 = local read "黄灯"() -> (w1409:bool)
        n853 = Not(x=w1407) -> (.not. x?=w1412:bool)
        n854 = Less?(x=w1415, y=1000.0) -> (x < y?=w1413:bool)
        n855 = Compound Arithmetic op=AND(w1408, w1412, w1409, w1413) -> (w1410:bool)
        n856 = case shown="真" w1410 {
          frame False {
          }
          frame True {
            n857 = flat-sequence {
              tunnel: [w1419] -> w1417
              tunnel: w1417 -> [w1421]
              tunnel: [w1421] -> w1416
              tunnel: w1416 -> [w1432]
              frame #0 {
                n858 = local read "电动缸电机"() -> (w1418:u32)
                n859 = call "PCI1220U运行.vi"("方向"=enum32{"Negative", "Positive"}."Positive" ("Direction"), "AxisHandle IN"=w1418) -> ("AxisHandle OUT"=w1419:u32)  [unwired: 9 in]
              }
              frame #1 {
                n860 = while {
                  stop <- w1429 stop-if-true
                  n861 = local read "电动缸前进"() -> (w1426:bool)
                  n862 = local read "齿条推拉力(N)"() -> (w1423:dbl)
                  n863 = Wait (ms)(milliseconds to wait=u32 50 ("毫秒倍数")) -> ()  [unwired: 1 out]
                  n864 = Absolute Value(x=w1423) -> (abs(x)=w1425:dbl)
                  n865 = local read "红灯"() -> (w1427:bool)
                  n866 = local read "复位"() -> (w1428:bool)
                  n867 = Greater?(x=w1425, y=1000.0) -> (0:w1422:bool)
                  n868 = Not(x=w1426) -> (.not. x?=w1430:bool)
                  n869 = Compound Arithmetic op=OR(w1428, w1427, w1430, w1422) -> (w1429:bool)
                }
              }
              frame #2 {
                n870 = call "PCI1220U停止.vi"("AxisHandle IN"=w1432) -> ()  [unwired: 9 in, 2 out]
              }
            }
          }
        }
      }
      frame #8 {
        n871 = local read "电动缸前进"() -> (w1433:bool)
        n872 = local read "齿条推拉力(N)"() -> (w1437:dbl)
        n873 = local read "电动缸后退"() -> (w1434:bool)
        n874 = Absolute Value(x=w1437) -> (abs(x)=w1441:dbl)
        n875 = local read "黄灯"() -> (w1435:bool)
        n876 = Not(x=w1433) -> (.not. x?=w1438:bool)
        n877 = Less?(x=w1441, y=1000.0) -> (x < y?=w1439:bool)
        n878 = Compound Arithmetic op=AND(w1434, w1438, w1435, w1439) -> (w1436:bool)
        n879 = case shown="真" w1436 {
          frame False {
          }
          frame True {
            n880 = flat-sequence {
              tunnel: [w1445] -> w1443
              tunnel: w1443 -> [w1447]
              tunnel: [w1447] -> w1442
              tunnel: w1442 -> [w1458]
              frame #0 {
                n881 = local read "电动缸电机"() -> (w1444:u32)
                n882 = call "PCI1220U运行.vi"("方向"=enum32{"Negative", "Positive"}."Negative" ("Direction"), "AxisHandle IN"=w1444) -> ("AxisHandle OUT"=w1445:u32)  [unwired: 9 in]
              }
              frame #1 {
                n883 = while {
                  stop <- w1455 stop-if-true
                  n884 = local read "电动缸后退"() -> (w1452:bool)
                  n885 = local read "齿条推拉力(N)"() -> (w1451:dbl)
                  n886 = Wait (ms)(milliseconds to wait=u32 50 ("毫秒倍数")) -> ()  [unwired: 1 out]
                  n887 = Absolute Value(x=w1451) -> (abs(x)=w1449:dbl)
                  n888 = local read "红灯"() -> (w1454:bool)
                  n889 = local read "复位"() -> (w1453:bool)
                  n890 = Greater?(x=w1449, y=1000.0) -> (0:w1448:bool)
                  n891 = Not(x=w1452) -> (.not. x?=w1456:bool)
                  n892 = Compound Arithmetic op=OR(w1453, w1454, w1456, w1448) -> (w1455:bool)
                }
              }
              frame #2 {
                n893 = call "PCI1220U停止.vi"("AxisHandle IN"=w1458) -> ()  [unwired: 9 in, 2 out]
              }
            }
          }
        }
      }
      frame #9 {
        n894 = local read "测头机构轴后退"() -> (w1459:bool)
        n895 = local read "测头机构轴前进"() -> (w1460:bool)
        n896 = local read "黄灯"() -> (w1461:bool)
        n897 = Not(x=w1459) -> (.not. x?=w1463:bool)
        n898 = Compound Arithmetic op=AND(w1460, w1463, w1461) -> (w1462:bool)
        n899 = case shown="真" w1462 {
          frame False {
          }
          frame True {
            n900 = flat-sequence {
              tunnel: [w1467] -> w1465
              tunnel: w1465 -> [w1469]
              tunnel: [w1469] -> w1464
              tunnel: w1464 -> [w1476]
              frame #0 {
                n901 = local read "测头机构电机"() -> (w1466:u32)
                n902 = call "PCI1220U运行.vi"("方向"=enum32{"Negative", "Positive"}."Positive" ("Direction"), "AxisHandle IN"=w1466) -> ("AxisHandle OUT"=w1467:u32)  [unwired: 9 in]
              }
              frame #1 {
                n903 = while {
                  stop <- w1473 stop-if-true
                  n904 = local read "测头机构轴前进"() -> (w1470:bool)
                  n905 = Wait (ms)(milliseconds to wait=u32 50 ("毫秒倍数")) -> ()  [unwired: 1 out]
                  n906 = local read "红灯"() -> (w1471:bool)
                  n907 = local read "复位"() -> (w1472:bool)
                  n908 = Not(x=w1470) -> (.not. x?=w1474:bool)
                  n909 = Compound Arithmetic op=OR(w1472, w1471, w1474) -> (w1473:bool)
                }
              }
              frame #2 {
                n910 = call "PCI1220U停止.vi"("AxisHandle IN"=w1476) -> ()  [unwired: 9 in, 2 out]
              }
            }
          }
        }
      }
      frame #10 {
        n911 = local read "测头机构轴前进"() -> (w1477:bool)
        n912 = local read "测头机构轴后退"() -> (w1478:bool)
        n913 = local read "黄灯"() -> (w1479:bool)
        n914 = Not(x=w1477) -> (.not. x?=w1481:bool)
        n915 = Compound Arithmetic op=AND(w1478, w1481, w1479) -> (w1480:bool)
        n916 = case shown="真" w1480 {
          frame False {
          }
          frame True {
            n917 = flat-sequence {
              tunnel: [w1485] -> w1483
              tunnel: w1483 -> [w1487]
              tunnel: [w1487] -> w1482
              tunnel: w1482 -> [w1494]
              frame #0 {
                n918 = local read "测头机构电机"() -> (w1484:u32)
                n919 = call "PCI1220U运行.vi"("方向"=enum32{"Negative", "Positive"}."Negative" ("Direction"), "AxisHandle IN"=w1484) -> ("AxisHandle OUT"=w1485:u32)  [unwired: 9 in]
              }
              frame #1 {
                n920 = while {
                  stop <- w1491 stop-if-true
                  n921 = local read "测头机构轴后退"() -> (w1488:bool)
                  n922 = Wait (ms)(milliseconds to wait=u32 50 ("毫秒倍数")) -> ()  [unwired: 1 out]
                  n923 = local read "红灯"() -> (w1490:bool)
                  n924 = local read "复位"() -> (w1489:bool)
                  n925 = Not(x=w1488) -> (.not. x?=w1492:bool)
                  n926 = Compound Arithmetic op=OR(w1489, w1490, w1492) -> (w1491:bool)
                }
              }
              frame #2 {
                n927 = call "PCI1220U停止.vi"("AxisHandle IN"=w1494) -> ()  [unwired: 9 in, 2 out]
              }
            }
          }
        }
      }
    }
    n928 = Wait (ms)(milliseconds to wait=u32 50 ("毫秒倍数")) -> ()  [unwired: 1 out]
    n929 = local read "停止"() -> (w1281:bool)
  }
  n930 = flat-sequence {
    tunnel: [w1498] -> w2
    tunnel: [w1496] -> w1
    tunnel: w2 -> [w1508]
    tunnel: w1 -> [w1507]
    frame #0 {
      n931 = First Call?() -> (First Call?: T/F=w1495:bool)
      n932 = case shown="真" w1495 {
        frame False {
        }
        frame True {
          n933 = while {
            i -> [w1502]
            stop <- w1503 stop-if-true
            w1506 = TRUE ("电动缸使能")
            n934 = Wait Until Next ms Multiple(millisecond multiple=u32 50 ("毫秒倍数")) -> ()  [unwired: 1 out]
            n935 = local write "回零完成"(FALSE ("回零完成")) -> ()
            n936 = local write "测头机构轴使能"(w1506) -> ()
            n937 = local write "旋转齿条轴使能"(w1506) -> ()
            n938 = local write "电动缸使能"(w1506) -> ()
            n939 = Greater Or Equal?(x=w1502, y=u32 30) -> (x >= y?=w1503:bool)
          }
        }
      }
      n940 = call "ADO Connection Create.vi"() -> ("error out"=w1499:errorcluster, "ADODB._Connection Out"=w1500:refnum<k7>)  [unwired: 10 in]
      n941 = call "ADO Connection Open.vi"("error in (no error)"=w1499, "ConnectionString"="Provider=Microsoft.Jet.OLEDB.4.0;Data Source=D:\\Q14070-Z060人机界面\\参数\\参数Z060.mdb;Persist Security Info=False;Jet OLEDB:Database Password=123;", "ADODB._Connection In"=w1500) -> ("error out"=w1496:errorcluster, "ADODB._Connection Out"=w1498:refnum<k7>)  [unwired: 7 in]
    }
    frame #1 {
      n942 = while {
        tunnel: w1508 -> [w1510]
        tunnel: w1507 -> [w1509]
        stop <- w1514 stop-if-true
        n943 = Wait (ms)(milliseconds to wait=u32 50 ("等待时间（毫秒）")) -> ()  [unwired: 1 out]
        n944 = First Call?() -> (First Call?: T/F=w1513:bool)
        n945 = Or(x=w1513, y="参数加载") -> (x .or. y?=w1512:bool)
        n946 = case shown="真" w1512 {
          tunnel: w1510 -> [_ w1517]
          tunnel: w1509 -> [_ w1516]
          frame False {
          }
          frame True {
            n947 = stacked-sequence {
              tunnel: w1517 -> [w1523 w1572 w1591]
              tunnel: w1516 -> [w1518 _ _]
              frame #0 {
                n948 = call "SQL Execute.vi"("error in (no error)"=w1518, "Command Text"="SELECT * FROM 测试参数表", "ADODB._Connection In"=w1523) -> ("Data"=w1521:string[][])  [unwired: 5 in, 3 out]
                n949 = Index Array(array=w1521, index (col)=0 ("索引 (行)")) -> (element=w1525:string[])  [unwired: 1 in]
                n950 = Array Size(array=w1525) -> (size(s)=w1520:i32)
                "型号数量" <- w1520
                n951 = while {
                  shift-right: [w1532] -> w1524
                  shift-left: i32[] [] -> [w1531]
                  tunnel: w1520 -> [w1529]
                  i -> [w1530]
                  stop <- w1528 stop-if-true
                  n952 = Greater Or Equal?(x=w1530, y=w1529) -> (x >= y?=w1528:bool)
                  n953 = Build Array (concatenate)(w1531, w1530) -> (w1532:i32[])
                }
                n954 = Build Cluster Array "索引与捆绑簇数组"(w1525, w1524) -> (w1519:cluster{"String":string, i32}[])
                n955 = property on="型号选择" class="Ring (严格)"("StringsAndValues[]"=w1519) -> ()  [unwired: 2 in, 2 out]
              }
              frame #1 {
                n956 = property on="型号选择" class="Ring (严格)"() -> ("RingText.Text"=w1573:string)  [unwired: 2 in, 2 out]
                n957 = call "创建文本2"("型号选择"=w1573) -> ("Result"=w1577:string)  [unwired: 13 in, 1 out]
                n958 = call "SQL Execute.vi"("Command Text"=w1577, "ADODB._Connection In"=w1572) -> ("Data"=w1576:string[][])  [unwired: 6 in, 3 out]
                n959 = Index Array(array=w1576, index (row)=0 ("索引 (行)")) -> (element=w1574:string[])  [unwired: 1 in]
                n960 = Fract/Exp String To Number ("分数/指数字符串至数值转换")(string=w1574) -> (number=w1561:dbl[])  [unwired: 3 in, 1 out]
                n961 = Index Array ("索引数组")(array=w1561, index #1=2 ("索引"), index #2=3 ("索引"), index #3=4 ("索引"), index #4=5 ("索引"), index #5=6 ("索引"), index #6=7 ("索引"), index #7=8 ("索引"), index #8=9 ("索引"), index #9=10 ("索引"), index #10=11 ("索引"), index #11=12 ("索引"), index #12=13 ("索引"), index #13=14 ("索引"), index #14=15 ("索引"), index #15=16 ("索引"), index #16=17 ("索引"), index #17=18 ("索引"), index #18=19 ("索引"), index #19=20 ("索引")) -> (element #1=w1560:dbl, element #2=w1559:dbl, element #3=w1558:dbl, element #4=w1557:dbl, element #5=w1556:dbl, element #6=w1555:dbl, element #7=w1554:dbl, element #8=w1553:dbl, element #9=w1552:dbl, element #10=w1551:dbl, element #11=w1550:dbl, element #12=w1549:dbl, element #13=w1543:dbl, element #14=w1542:dbl, element #15=w1541:dbl, element #16=w1540:dbl, element #17=w1536:dbl, element #18=w1535:dbl, element #19=w1533:dbl)
                n962 = local write "测头机构轴移动速度"(w1560) -> ()
                n963 = local write "测头机构轴检测位"(w1559) -> ()
                n964 = local write "测头机构轴后退位"(w1557) -> ()
                n965 = local write "测头机构轴待检位"(w1558) -> ()
                n966 = local write "旋转伺服找帽转速"(w1553) -> ()
                n967 = local write "旋转伺服测量转速"(w1552) -> ()
                n968 = local write "总行程标准(mm)"(w1550) -> ()
                n969 = local write "齿条移动速度"(w1556) -> ()
                n970 = local write "平均轴向力MAX(N)"(w1540) -> ()
                n971 = local write "最大轴向力标准(N)"(w1543) -> ()
                n972 = local write "齿条左极限"(w1555) -> ()
                n973 = local write "总行程最大值"(w1549) -> ()
                n974 = local write "齿条右极限"(w1554) -> ()
                n975 = local write "转向器中心"(w1533) -> ()
                n976 = local write "总圈数标准"(w1536) -> ()
                n977 = local write "总圈数最大值"(w1535) -> ()
                n978 = local write "测量点扭矩"(w1551) -> ()
                n979 = local write "力波动标准(N)"(w1542) -> ()
                n980 = local write "轴向力标准(N)"(w1541) -> ()
              }
              frame #2 {
                n981 = call "SQL Execute.vi"("Command Text"="SELECT * FROM 传感器校验表 where ID='1'", "ADODB._Connection In"=w1591) -> ("Data"=w1593:string[][])  [unwired: 6 in, 3 out]
                n982 = Index Array(array=w1593) -> (element=w1594:string[])  [unwired: 2 in]
                n983 = Fract/Exp String To Number ("分数/指数字符串至数值转换")(string=w1594) -> (number=w1584:dbl[])  [unwired: 3 in, 1 out]
                n984 = Index Array(array=w1584, index #1=1 ("索引"), index #2=2 ("索引"), index #3=3 ("索引"), index #4=4 ("索引"), index #5=5 ("索引"), index #6=6 ("索引")) -> (element #1=w1583:dbl, element #2=w1582:dbl, element #3=w1581:dbl, element #4=w1580:dbl, element #5=w1579:dbl, element #6=w1578:dbl)
                n985 = local write "间隙位移零点偏移"(w1583) -> ()
                n986 = local write "间隙位移比例偏移"(w1582) -> ()
                n987 = local write "齿条推拉力零点偏移"(w1581) -> ()
                n988 = local write "齿条推拉力比例偏移"(w1580) -> ()
                n989 = local write "齿条扭矩零点偏移"(w1579) -> ()
                n990 = local write "齿条扭矩比例偏移"(w1578) -> ()
              }
            }
          }
        }
        n991 = local read "停止"() -> (w1514:bool)
        "ADODB._Connection Out 2" <- w1510
      }
    }
  }
  n992 = while {
    stop <- w1596 stop-if-true
    n993 = local read "rfid工步号"() -> (w1595:u32)
    n994 = case shown="10" w1595 {
      frame 0, Default {
      }
      frame 10 {
        n995 = flat-sequence {
          tunnel: [w1606] -> w1600
          tunnel: w1600 -> [w1610]
          tunnel: [w1607] -> w1599
          tunnel: w1599 -> [w1612]
          tunnel: [w1612] -> w1598
          tunnel: w1598 -> [w1615]
          frame #0 {
            n996 = while {
              stop <- w1601 stop-if-true
              n997 = local read "rfid触发"() -> (w1601:bool)
              n998 = Wait Until Next ms Multiple(millisecond multiple=u32 50 ("毫秒倍数")) -> ()  [unwired: 1 out]
            }
          }
          frame #1 {
            n999 = local write "芯片ID"("" ("随行板ID")) -> ()
            n1000 = local write "rfid完成"(FALSE ("RFID完成")) -> ()
            n1001 = local write "rfid触发"(FALSE ("RFID读取触发")) -> ()
          }
          frame #2 {
            n1002 = local read "Z060ARFID"() -> (w1606:string)
            n1003 = local write "芯片ID"(w1606) -> ()
          }
          frame #3 {
            w1608 = T6 0 items=["两端", "字符串首端", "字符串末端"] ("location (both)")
            n1004 = call "查询产品ID.vi"("芯片编码"=w1610) -> ("产品ID"=w1609:string)  [unwired: 8 in, 2 out]
            "读取产品ID" <- w1609
            n1005 = call <vilib>:"Trim Whitespace.vi"("string"=w1609, "location (both)"=w1608) -> ("trimmed string"=w1607:string)
          }
          frame #4 {
            n1006 = Wait Until Next ms Multiple(millisecond multiple=u32 500 ("毫秒倍数")) -> ()  [unwired: 1 out]
          }
          frame #5 {
            n1007 = call "查询上序合格.vi"("产品ID"=w1615) -> ("本序已做"=w1613:bool, "上序合格"=w1614:bool)  [unwired: 8 in, 1 out]
            n1008 = Not(x=w1614) -> (.not. x?=w1616:bool)
            n1009 = local write "上序不合格"(w1616) -> ()
            n1010 = local write "上序合格"(w1614) -> ()
            n1011 = local write "本序已做"(w1613) -> ()
          }
          frame #6 {
            n1012 = local write "rfid完成"(TRUE ("RFID读取完成")) -> ()
            n1013 = Wait Until Next ms Multiple(millisecond multiple=u32 500 ("毫秒倍数")) -> ()  [unwired: 1 out]
          }
          frame #7 {
            "rfid工步号" <- 15.0 ("工步号")
          }
        }
      }
      frame 210 {
        n1014 = local read "读取产品ID"() -> (w1620:string)
        n1015 = local write "产品ID"(w1620) -> ()
      }
    }
    n1016 = Wait Until Next ms Multiple(millisecond multiple=u32 50 ("毫秒倍数")) -> ()  [unwired: 1 out]
    n1017 = local read "停止"() -> (w1596:bool)
  }
  n1018 = flat-sequence {
    tunnel: [w1621] -> w4
    tunnel: w4 -> [w1627]
    tunnel: [w1626] -> w3
    tunnel: w3 -> [w1697]
    frame #0 {
      n1019 = call "PCI1240U初始化.vi"() -> ("旋转电机"=→"旋转齿条电机":u32, "电动缸电机"=→"电动缸电机":u32, "DeviceHandle"=→"DeviceHandle":u32, "进给电机"=→"测头机构电机":u32)  [unwired: 6 in, 2 out]
      n1020 = call "PCI8622配置.vi"() -> ("DeviceID"=w1621:i32)  [unwired: 11 in]
    }
    frame #1 {
      n1021 = while {
        tunnel: w1627 -> [w1629]
        tunnel: [w1628] -> w1626
        stop <- "停止" stop-if-true
        n1022 = stacked-sequence {
          tunnel: w1629 -> [_ _ w1673]
          tunnel: [_ _ w1673] -> w1628
          frame #0 {
            n1023 = local read "测头机构电机"() -> (w1638:u32)
            n1024 = Boolean To (0,1)(Boolean="测头机构轴使能") -> (0, 1=w1636:i16)
            n1025 = call <userlib>:"Acm_AxSetSvOn.vi"("OnOff"=w1636, "AxisHandle"=w1638) -> ("AxisHandle"=w1635:u32)  [unwired: 1 in, 2 out]
            n1026 = call "PCI1220U进给轴速度设置.vi"("Change Velocity"="测头机构轴速度(mm/s)", "AxisHandle IN"=w1635) -> ("AxisHandle OUT"=w1633:u32)  [unwired: 9 in]
            n1027 = call "PCI1220U进给轴读取位置.vi"("AxisHandle IN"=w1633) -> ("位置"=→"测头机构轴位置(mm)":dbl)  [unwired: 9 in, 1 out]
          }
          frame #1 {
            n1028 = local read "电动缸电机"() -> (w1648:u32)
            n1029 = local read "旋转齿条电机"() -> (w1647:u32)
            n1030 = Boolean To (0,1)(Boolean="电动缸使能") -> (0, 1=w1652:i16)
            n1031 = Boolean To (0,1)(Boolean="旋转齿条轴使能") -> (0, 1=w1646:i16)
            n1032 = call <userlib>:"Acm_AxSetSvOn.vi"("OnOff"=w1646, "AxisHandle"=w1647) -> ("AxisHandle"=w1649:u32)  [unwired: 1 in, 2 out]
            n1033 = call <userlib>:"Acm_AxSetSvOn.vi"("OnOff"=w1652, "AxisHandle"=w1648) -> ("AxisHandle"=w1651:u32)  [unwired: 1 in, 2 out]
            n1034 = call "PCI1220U扭矩轴速度设置.vi"("Change Velocity"="旋转伺服速度(°/s)", "AxisHandle IN"=w1649) -> ("AxisHandle OUT"=w1650:u32)  [unwired: 9 in]
            n1035 = call "PCI1240电动缸速度设置.vi"("Change Velocity"="电动缸速度(mm/s)", "AxisHandle IN"=w1651) -> ("AxisHandle OUT"=w1639:u32)  [unwired: 9 in]
            n1036 = call "PCI1220U扭矩轴读取位置.vi"("AxisHandle IN"=w1650) -> ("位置"=→"旋转伺服位置(°)":dbl)  [unwired: 9 in, 1 out]
            n1037 = call "PCI1240电动缸读取位置.vi"("AxisHandle IN"=w1639) -> ("位置"=→"电动缸位置(mm)":dbl)  [unwired: 9 in, 1 out]
          }
          frame #2 {
            w1689 = 0  # nRetSizeWords
            w1690 = 2048  # nReadSizeWords
            # "hDevice"
            n1038 = Initialize Array(u16 0, 2048 ("dimension size")) -> (w1680:u16[])
            n1039 = dll-call lib="PCI8622_32.dll" fn="PCI8622_ReadDeviceProAD_Npt" label="ReadDeviceProAD_Npt"("hDevice"=w1673, "ADBuffer[]"=w1680, "nReadSizeWords"=w1690, "nRetSizeWords"=w1689) -> ("ADBuffer[]"=w1683:u16[])  [unwired: 7 in, 2 out]
            n1040 = Divide(x=w1683, y=65536.01) -> (x/y=w1684:dbl[])
            n1041 = Multiply(x=w1684, y=20) -> (x*y=w1687:dbl[])
            n1042 = Subtract(x=w1687, y=10) -> (x-y=w1679:dbl[])
            n1043 = Decimate 1D Array ("抽取一维数组")(w1679) -> (w1667:dbl[], w1668:dbl[], w1666:dbl[])  [unwired: 5 out]
            n1044 = Add Array Elements(numeric array=w1667) -> (sum=w1676:dbl)
            n1045 = Add Array Elements(numeric array=w1666) -> (sum=w1677:dbl)
            n1046 = Array Size(array=w1667) -> (size(s)=w1675:i32)
            n1047 = Add Array Elements(numeric array=w1668) -> (sum=w1672:dbl)
            n1048 = Array Size(array=w1666) -> (size(s)=w1678:i32)
            n1049 = Array Size(array=w1668) -> (size(s)=w1674:i32)
            n1050 = Divide(x=w1676, y=w1675) -> (x/y=w1665:dbl)
            n1051 = Divide(x=w1677, y=w1678) -> (x/y=w1657:dbl)
            n1052 = Divide(x=w1672, y=w1674) -> (x/y=w1662:dbl)
            n1053 = Subtract(x=w1657, y=2.371) -> (x-y=w1655:dbl)
            n1054 = Multiply(x=w1665, y=2.0) -> (x*y=w1660:dbl)
            n1055 = Multiply(x=w1662, y=200.0) -> (x*y=w1661:dbl)
            n1056 = Subtract(x=w1660, y=-1.0) -> (x-y=w1658:dbl)
            n1057 = Multiply(x=w1655, y=0.75) -> (x*y=w1653:dbl)
            n1058 = local read "间隙位移比例偏移"() -> (w1694:dbl)
            n1059 = local read "间隙位移零点偏移"() -> (w1693:dbl)
            n1060 = local read "齿条扭矩零点偏移"() -> (w1695:dbl)
            n1061 = local read "齿条扭矩比例偏移"() -> (w1696:dbl)
            n1062 = local read "齿条推拉力比例偏移"() -> (w1692:dbl)
            n1063 = local read "齿条推拉力零点偏移"() -> (w1691:dbl)
            n1064 = call "传感器校订.vi"("零点"=w1695, "比例"=w1696, "传感器"=w1658) -> ("示值"=→"齿条扭矩(Nm)":dbl)  [unwired: 8 in]
            n1065 = call "传感器校订.vi"("零点"=w1693, "比例"=w1694, "传感器"=w1653) -> ("示值"=→"间隙位移(mm)":dbl)  [unwired: 8 in]
            n1066 = call "传感器校订.vi"("零点"=w1691, "比例"=w1692, "传感器"=w1661) -> ("示值"=→"齿条推拉力(N)":dbl)  [unwired: 8 in]
          }
        }
        n1067 = Wait Until Next ms Multiple(millisecond multiple=u32 50 ("毫秒倍数")) -> ()  [unwired: 1 out]
      }
    }
    frame #2 {
      n1068 = dll-call lib="PCI8622_32.dll" fn="PCI8622_StopDeviceProAD" label="StopDeviceProAD"("hDevice"=w1697) -> ("hDevice"=w1698:i32)  [unwired: 4 in, 2 out]
      n1069 = dll-call lib="PCI8622_32.dll" fn="PCI8622_ReleaseDeviceProAD" label="ReleaseDeviceProAD"("hDevice"=w1698) -> ()  [unwired: 5 in, 2 out]
      n1070 = dll-call lib="PCI8622_32.dll" fn="PCI8622_ReleaseDevice" label="ReleaseDevice"("hDevice"=w1697) -> ()  [unwired: 5 in, 2 out]
    }
  }
